vi "ADIS16448 Loop.vi"(8 "error in":errorcluster) -> ()   [LabVIEW 2019]
uses:
  Typedef/ADIS16448 Device Reference.ctl
  Typedef/ADIS16448 Hardware Configuration.ctl
  <vilib>/Rock Robotics/WPI/SPI/WPI_SPIMode.ctl
  <vilib>/Rock Robotics/SystemInterfaces/DIO/FPGA_DIOChannel.ctl
  <vilib>/Rock Robotics/SystemInterfaces/spilib/spi_bus.ctl
  Typedef/ADIS16448 Status.ctl
  Typedef/ADIS16448 Data.ctl
  Typedef/ADIS16448 Process.ctl
  Typedef/ADIS16448 Command Type.ctl
  <vilib>/Rock Robotics/SystemInterfaces/CounterEncoderSourceConvertion/FPGA_CounterEncoderSourceConvertionLVSourceType.ctl
  <vilib>/Rock Robotics/SystemInterfaces/DIO/FPGA_DIODigitalSourceChannel.ctl
  <vilib>/Rock Robotics/SystemInterfaces/AnalogTrigger/FPGA_AnalogTriggerIndex.ctl
  <vilib>/Rock Robotics/SystemInterfaces/AnalogTrigger/FPGA_AnalogTriggerOutType.ctl
  Typedef/ADIS16448 Loop State.ctl
  Typedef/ADIS16448 Loop Data.ctl
  <vilib>/Rock Robotics/WPI/SPI/WPI_SPIDevRef.ctl
  Typedef/ADIS16448 Register.ctl
  Typedef/ADIS16448 Call Buffer Cmd.ctl
  ADIS16448 Loop Update Globals.vi
  ADIS16448 Globals.vi
  <vilib>/Rock Robotics/WPI/Counter/WPI_CounterDigitalInputToDigitalSource.vi
  <vilib>/Rock Robotics/WPI/SPI/WPI_SPIWrite.vi
  <vilib>/Rock Robotics/WPI/SPI/WPI_SPIRead.vi
  <vilib>/Rock Robotics/WPI/ThirdParty/JAS_Junk/TrajLib/Trajectory_Library.lvlib
panel:
  in  "Use Register Read Mode":bool=TRUE
  in  "Calibration Time":i32
  in  "element":T1
  in  "ADIS16448DevRef":T2={"DevStatus"={"status"=FALSE, "code"=0, "source"=""}, "Hardware Config"={"SPI Clock Rate (Hz)"=1000000.0, "IMU SPI Mode (3)"=enum."Mode 3 (Clk Idle High,Sample on Trailing)", "IMU Reset Pin"=enum."SPI Port CS2", "IMU SPI Bus"=enum."SPI On-Board, CS0", "IMU Data Ready Pin"=enum."SPI Port CS1", "Stall Config"={"Pow2BytesPerRead"=255, "StallTicks"=640, "CsToSclkTicks"=5}, "IMU Status LED Pin"=enum."DIO MXP 9"}, "Calibration Complete"=refnum, "Status FIFO"=refnum, "Last Value Reference"=refnum, "Sychronous Process VI"=refnum, "Cmd FIFO"=refnum, "Source"={"DevStatus"={"status"=FALSE, "code"=0, "source"=""}, "AnalogTriggerMode?"=FALSE, "DigitalMode"={"DIO Channel"=enum."Disabled"}, "AnalogTriggerMode"={"AnalogTriggerIndex"=enum."Trig 0", "OutputType"=enum."InWindow"}}, "Data FIFO"=refnum, "IMU Status LED Pin"=enum."DIO MXP 9", "Calibration Time"=5}
  in  "Main Name":string
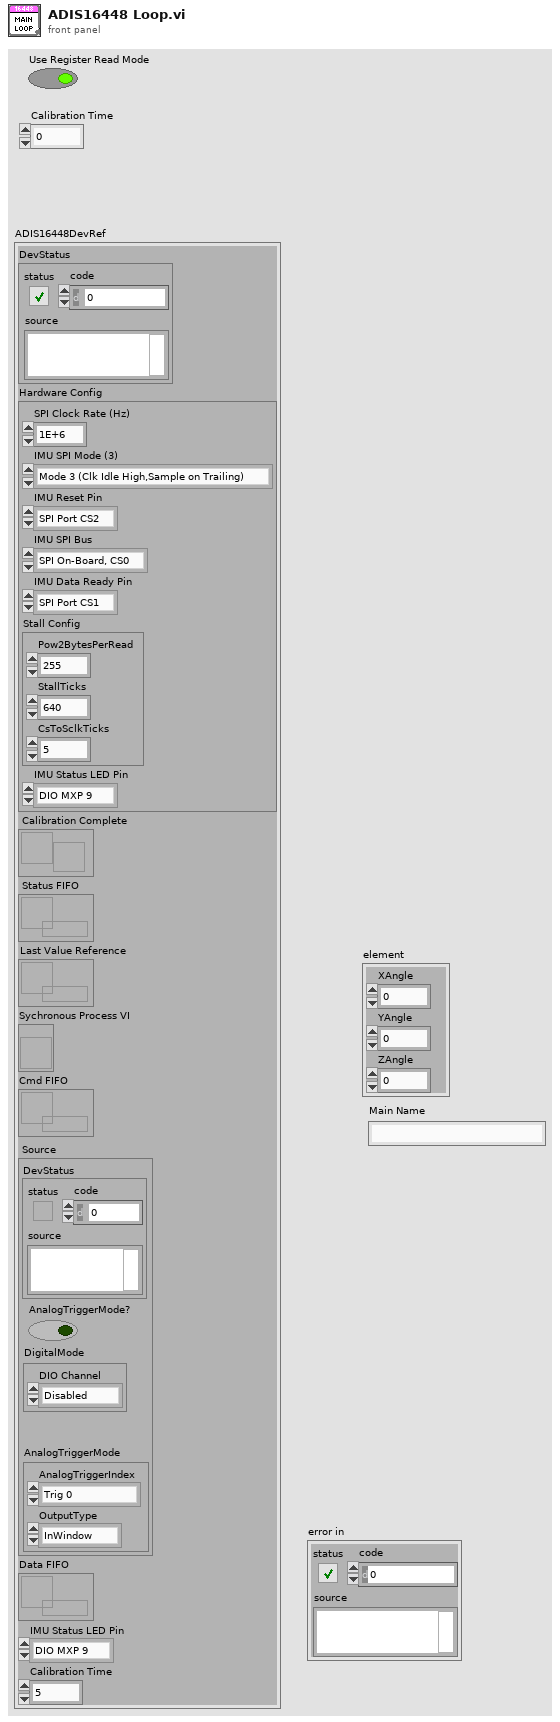
[diagram p1: front panel]
types:
  T1 = typedef "ADIS16448 Data.ctl" = cluster{"XAngle":dbl, "YAngle":dbl, "ZAngle":dbl}
  T2 = typedef "ADIS16448 Device Reference.ctl" = cluster{"DevStatus":errorcluster, "Hardware Config":T3, "Calibration Complete":refnum<notifier>, "Status FIFO":refnum<k33>, "Last Value Reference":refnum<data-value>, "Sychronous Process VI":T7, "Cmd FIFO":refnum<k33>, "Source":T8, "Data FIFO":refnum<k33>, "IMU Status LED Pin":T5, "Calibration Time":u32}
  T3 = typedef "ADIS16448 Hardware Configuration.ctl" = cluster{"SPI Clock Rate (Hz)":dbl, "IMU SPI Mode (3)":T4, "IMU Reset Pin":T5, "IMU SPI Bus":T6, "IMU Data Ready Pin":T5, "Stall Config":cluster{"Pow2BytesPerRead":u8, "StallTicks":u16, "CsToSclkTicks":u8}, "IMU Status LED Pin":T5}
  T4 = typedef "WPI_SPIMode.ctl" = enum16{"Mode 0 (Clk Idle Low,Sample on Leading)", "Mode 1 (Clk Idle Low,Sample on Trailing)", "Mode 2 (Clk Idle High,Sample on Leading)", "Mode 3 (Clk Idle High,Sample on Trailing)"}
  T5 = typedef "FPGA_DIOChannel.ctl" = enum8{"DIO 0", "DIO 1", "DIO 2", "DIO 3", "DIO 4", "DIO 5", "DIO 6", "DIO 7", "DIO 8", "DIO 9", "DIO MXP 0", "DIO MXP 1", "DIO MXP 2", "DIO MXP 3", "DIO MXP 4", "DIO MXP 5", "DIO MXP 6", "DIO MXP 7", "DIO MXP 8", "DIO MXP 9", "DIO MXP 10", "DIO MXP 11", "DIO MXP 12", "DIO MXP 13", "DIO MXP 14", "DIO MXP 15", "SPI Port CS1", "SPI Port CS2", "SPI Port CS3", "SPI Port MISO", "SPI Port MOSI", "Invalid"}
  T6 = typedef "spi_bus.ctl" = enum16{"SPI On-Board, CS0", "SPI On-Board, CS1", "SPI On-Board, CS2", "SPI On-Board, CS3", "SPI MXP", "Invalid"}
  T7 = typedef "ADIS16448 Process.ctl" = refnum<vi>
  T8 = typedef "FPGA_CounterEncoderSourceConvertionLVSourceType.ctl" = cluster{"DevStatus":errorcluster, "AnalogTriggerMode?":bool, "DigitalMode":cluster{"DIO Channel":T9}, "AnalogTriggerMode":cluster{"AnalogTriggerIndex":T10, "OutputType":T11}}
  T9 = typedef "FPGA_DIODigitalSourceChannel.ctl" = enum8{"DIO 0", "DIO 1", "DIO 2", "DIO 3", "DIO 4", "DIO 5", "DIO 6", "DIO 7", "DIO 8", "DIO 9", "DIO MXP 0", "DIO MXP 1", "DIO MXP 2", "DIO MXP 3", "DIO MXP 4", "DIO MXP 5", "DIO MXP 6", "DIO MXP 7", "DIO MXP 8", "DIO MXP 9", "DIO MXP 10", "DIO MXP 11", "DIO MXP 12", "DIO MXP 13", "DIO MXP 14", "DIO MXP 15", "SPI Port CS1", "SPI Port CS2", "SPI Port CS3", "SPI Port MISO", "SPI Port MOSI", "Disabled"}
  T10 = typedef "FPGA_AnalogTriggerIndex.ctl" = enum8{"Trig 0", "Trig 1", "Trig 2", "Trig 3", "Trig 4", "Trig 5", "Trig 6", "Trig 7", "Invalid"}
  T11 = typedef "FPGA_AnalogTriggerOutType.ctl" = enum16{"InWindow", "TriggerState", "Rising", "Falling"}
  T12 = typedef "ADIS16448 Register.ctl" = u8
  T13 = typedef "ADIS16448 Loop State.ctl" = enum16{"Default", "Error", "***Initialization***", "Reset", "Register DR Source", "Start SPI", "Write Config", "Init Auto SPI", "***Calibration***", "Calibrate", "Finish Cal", "***Operation***", "Run", "Process", "Run Cmds", "Run_Alt", "Run_Cmds_Alt", "Cal_Init_Alt", "Cal_Alt"}
  T14 = typedef "ADIS16448 Loop Data.ctl" = cluster{"SPIDevRef":T15, "Data Counter":u16, "Reset":bool, "Digital Source":T8, "Bytes Per Sample":u32, "Data":dbl[], "ADIS16448DevRef":T2, "TimeStampPrev":u32, "Sensor to Robot Rotation":dbl[][], "AutoSPI Active?":bool, "Offsets":dbl[], "Offset Counter":i32, "Data Header":u8[], "Zero Byte Count":u8, "Running Offset":dbl[], "CalSamplesAlt":i32, "CalCountAlt":i32}
  T15 = typedef "WPI_SPIDevRef.ctl" = cluster{"DevStatus":errorcluster, "Handle":i32, "SPI Bus":T6}
  T16 = typedef "ADIS16448 Status.ctl" = cluster{"Calibrated?":bool, "IMU Detected?":bool}
  T17 = typedef "ADIS16448 Call Buffer Cmd.ctl" = enum16{"Add Item ", "Calculate"}
  T18 = typedef "ADIS16448 Command Type.ctl" = cluster{"Command":enum16{"None", "Reset", "Rewrite Config", "Start Recal", "Recalibrate", "Recal Complete", "Exit Auto SPI", "Start Auto SPI", "Configure Cal"}, "Data":u32}
  T19 = typedef "WPI_DigitalOutputDevRef.ctl" = cluster{"DIO Channel":T5, "DevStatus":errorcluster}
  T20 = typedef "WPI_DigitalInputDevRef.ctl" = cluster{"DevStatus":errorcluster, "DIO Channel":T5}
  T21 = cluster{"Pow2BytesPerRead":u8, "StallTicks":u16, "CsToSclkTicks":u8}
  T22 = enum16{"None", "Reset", "Rewrite Config", "Start Recal", "Recalibrate", "Recal Complete", "Exit Auto SPI", "Start Auto SPI", "Configure Cal"}
  T23 = enum32{"Bad", "Idle", "Run top level", "Running"}
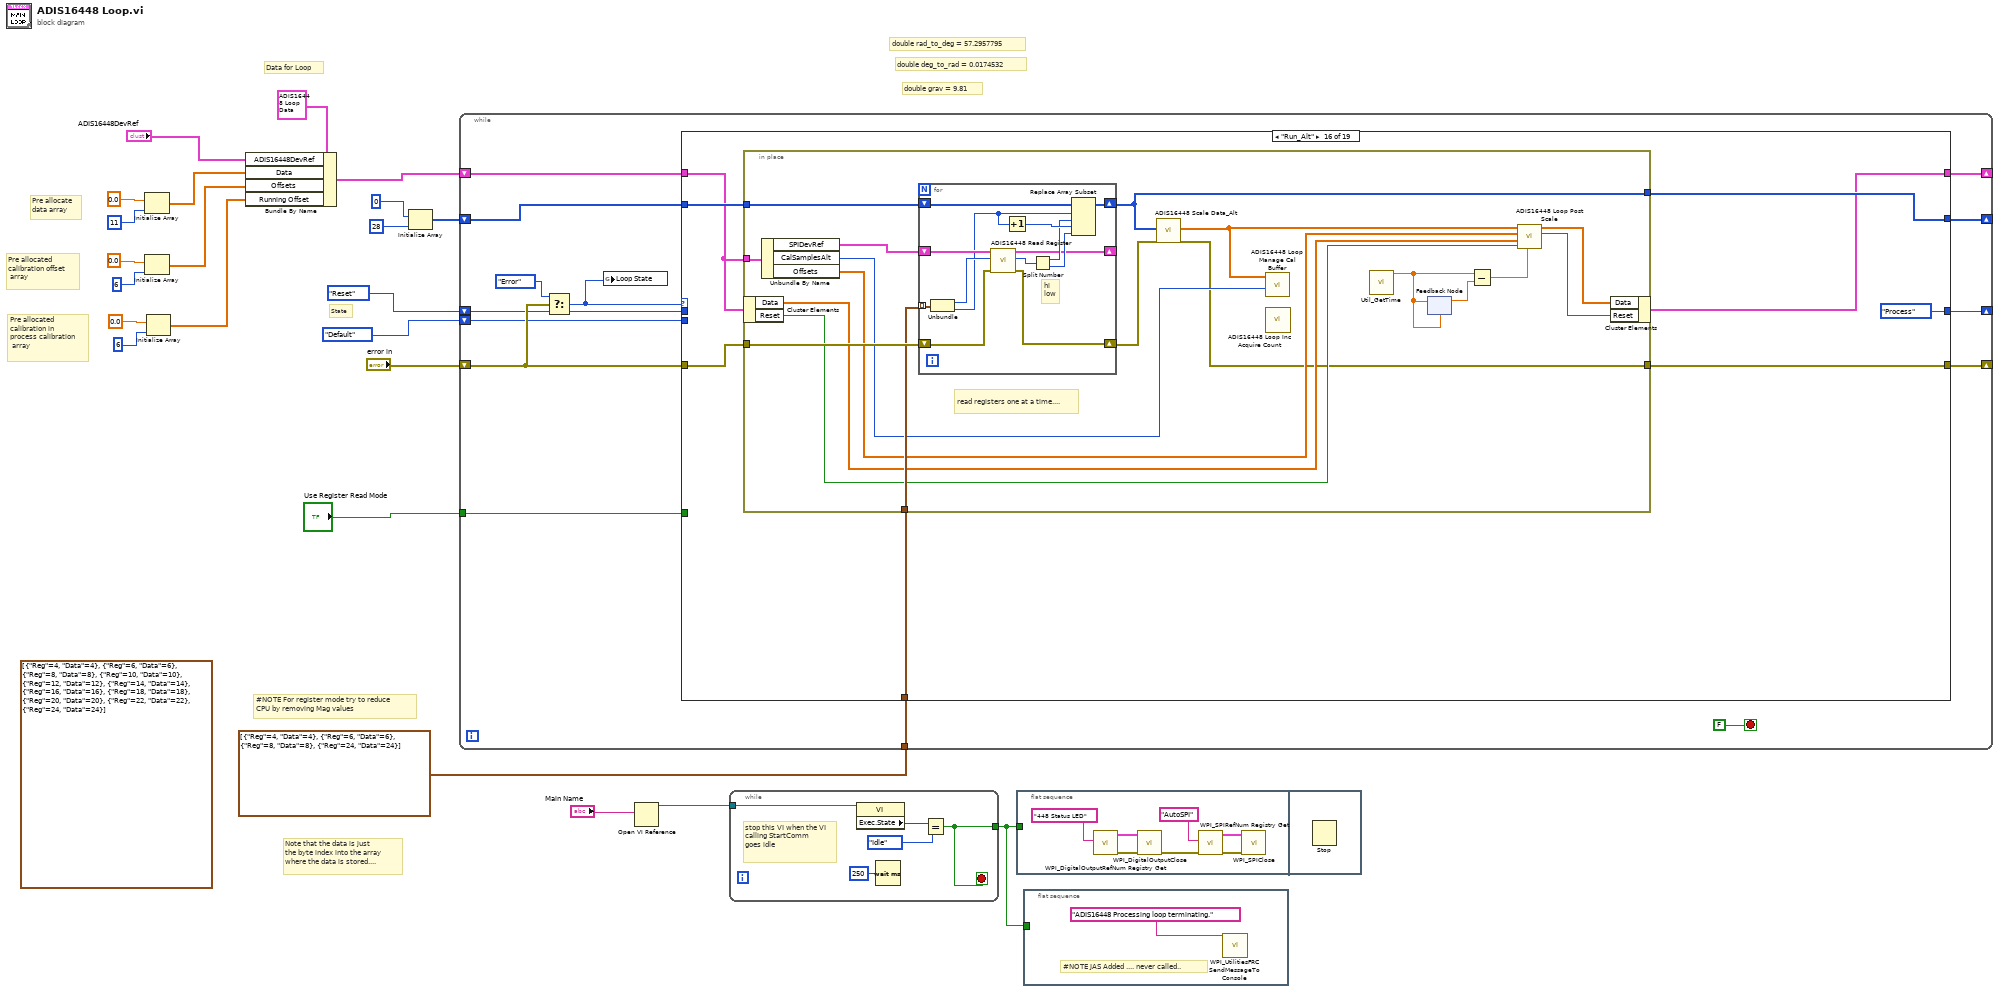
[diagram p0: block diagram]
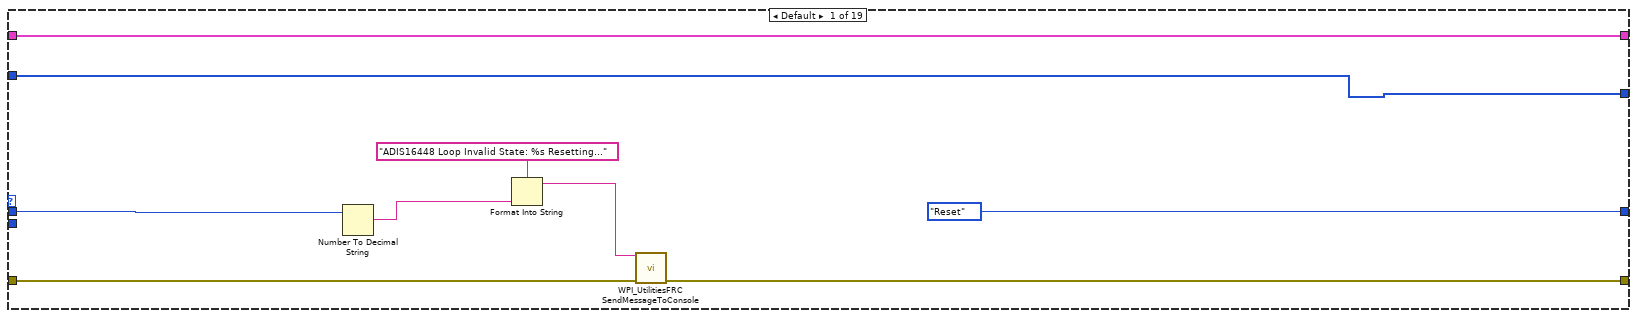
[diagram p2: hidden frame]
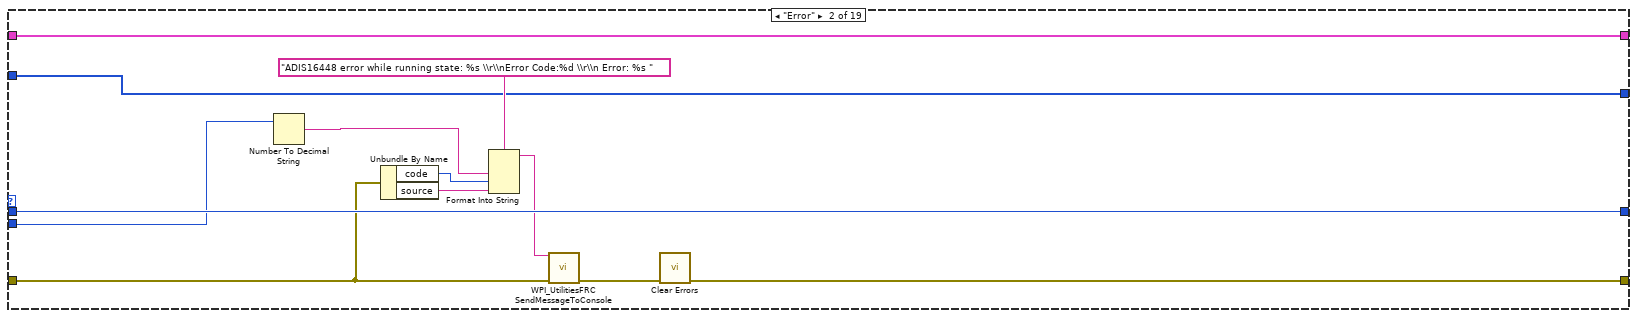
[diagram p3: hidden frame]
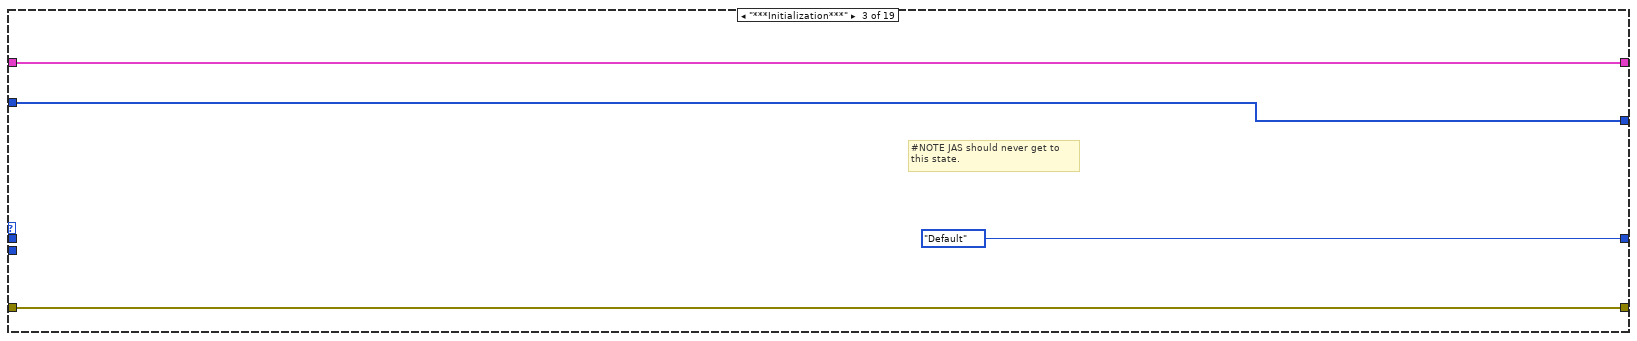
[diagram p4: hidden frame]
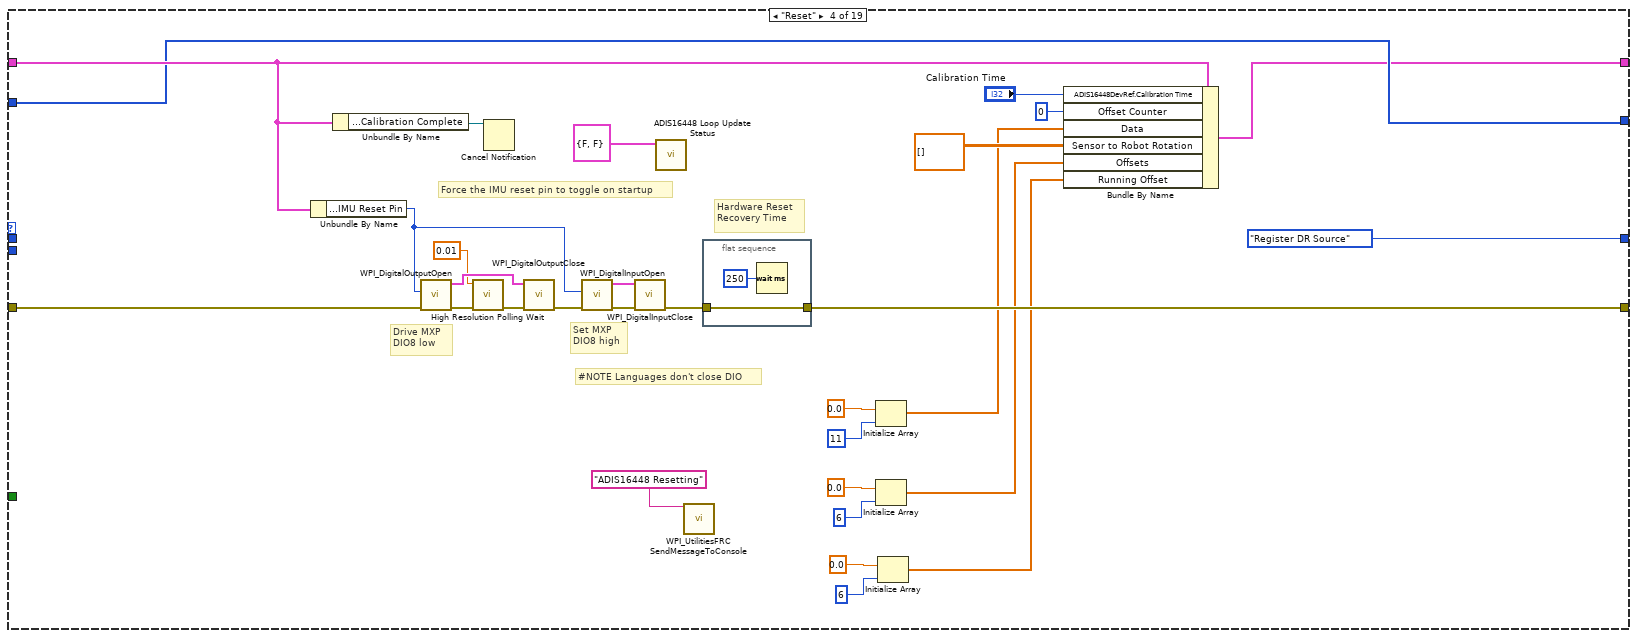
[diagram p5: hidden frame]
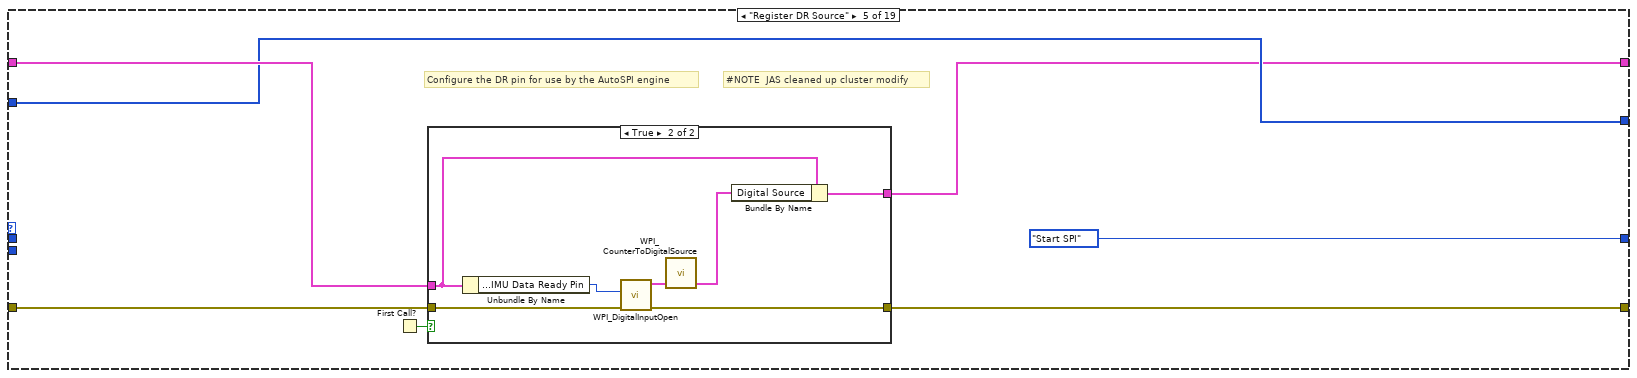
[diagram p6: hidden frame]
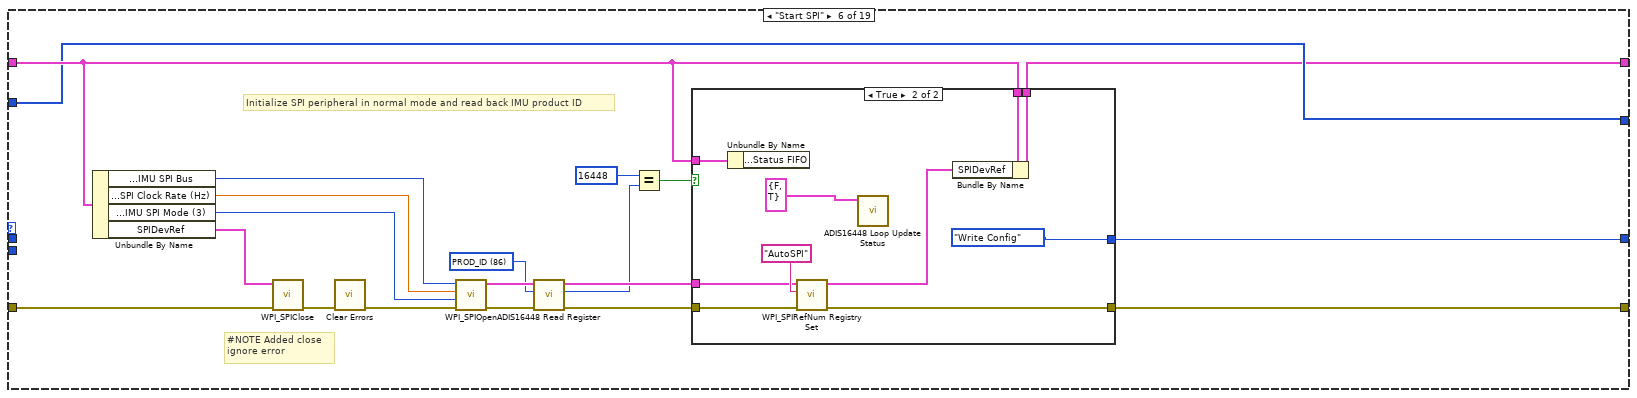
[diagram p8: hidden frame]
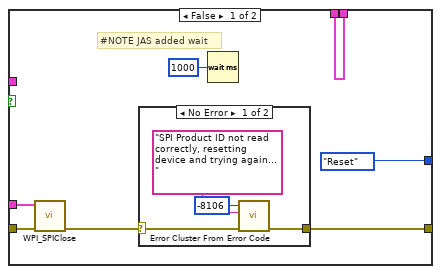
[diagram p9: hidden frame]
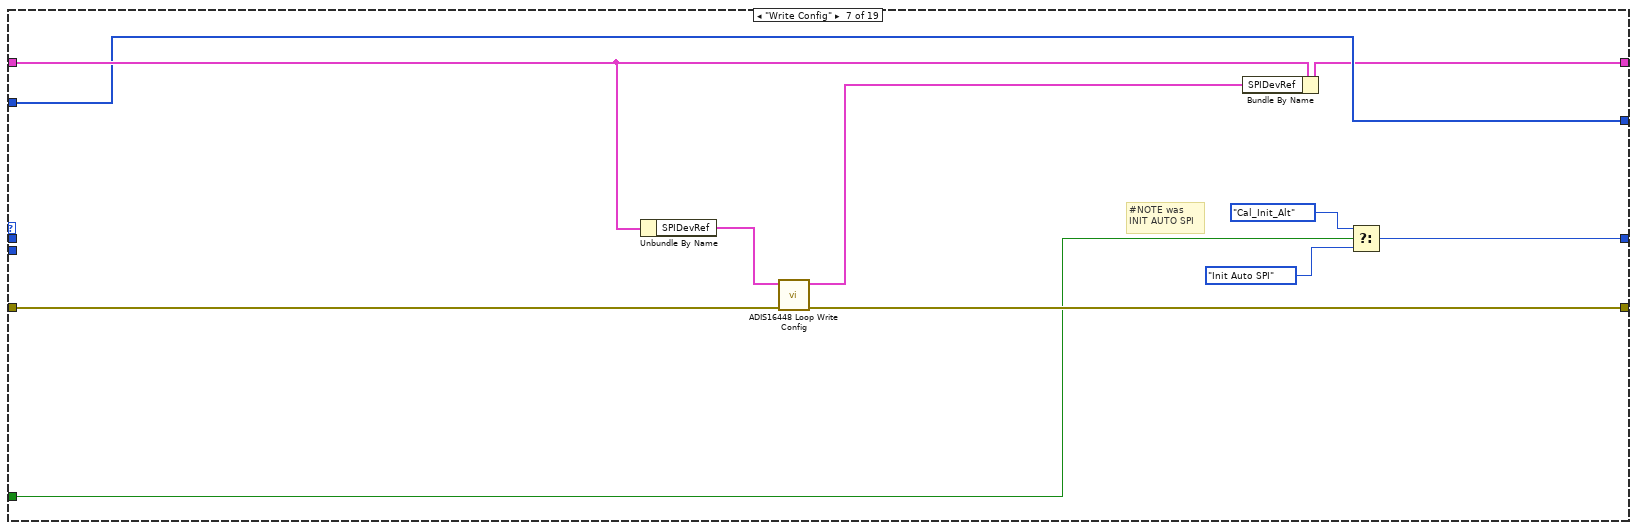
[diagram p11: hidden frame]
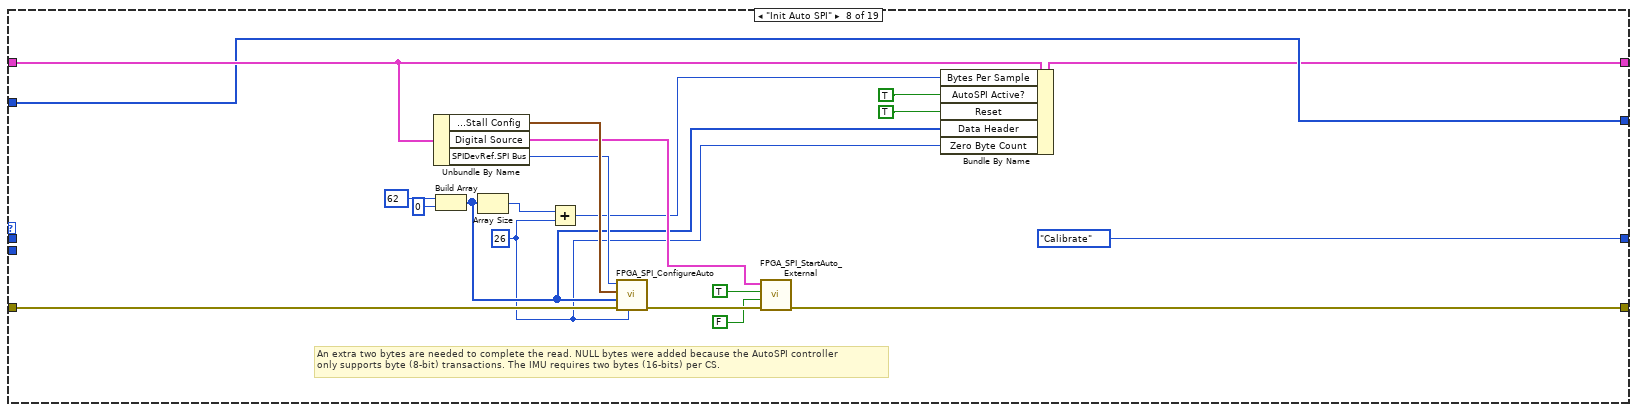
[diagram p12: hidden frame]
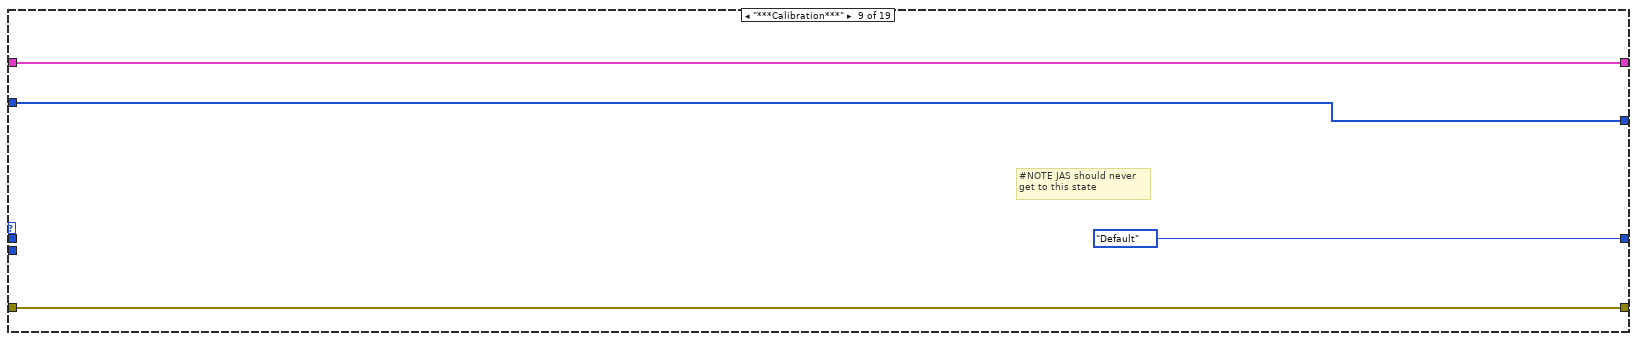
[diagram p13: hidden frame]
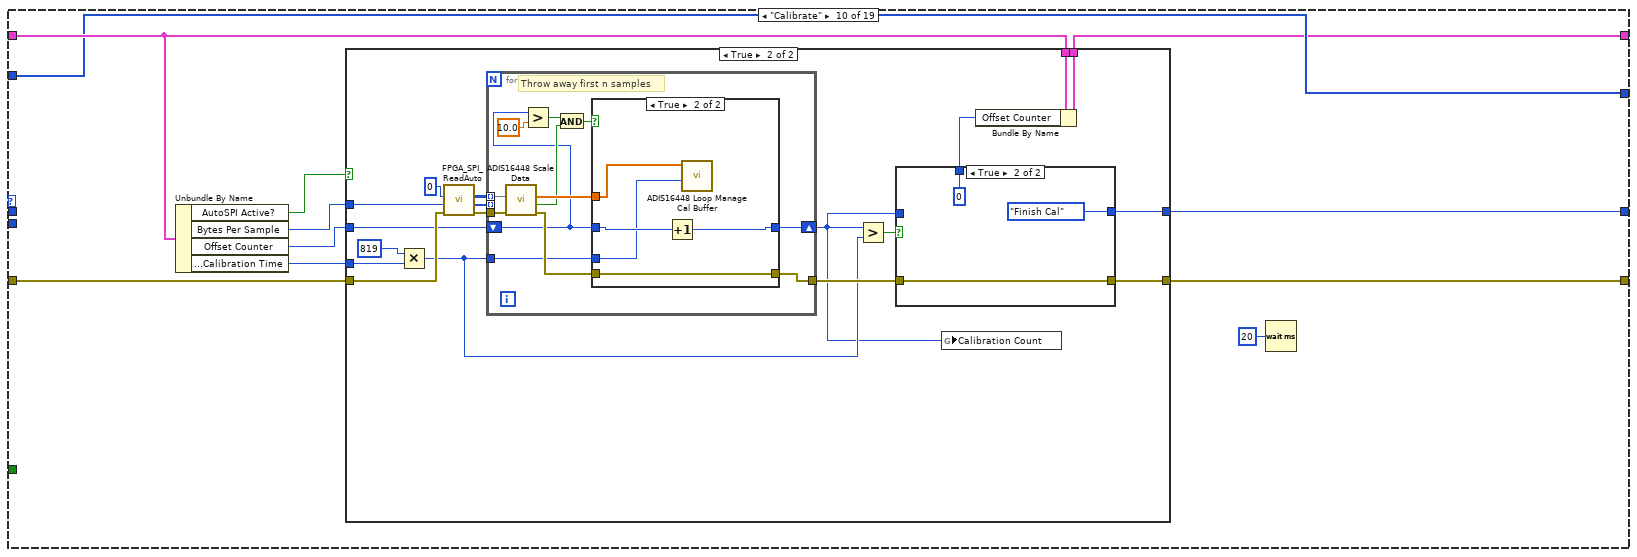
[diagram p14: hidden frame]
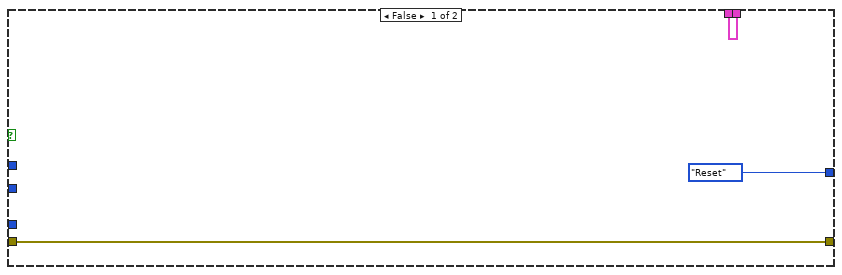
[diagram p15: hidden frame]
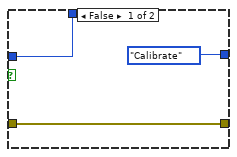
[diagram p16: hidden frame]
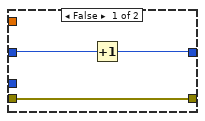
[diagram p17: hidden frame]
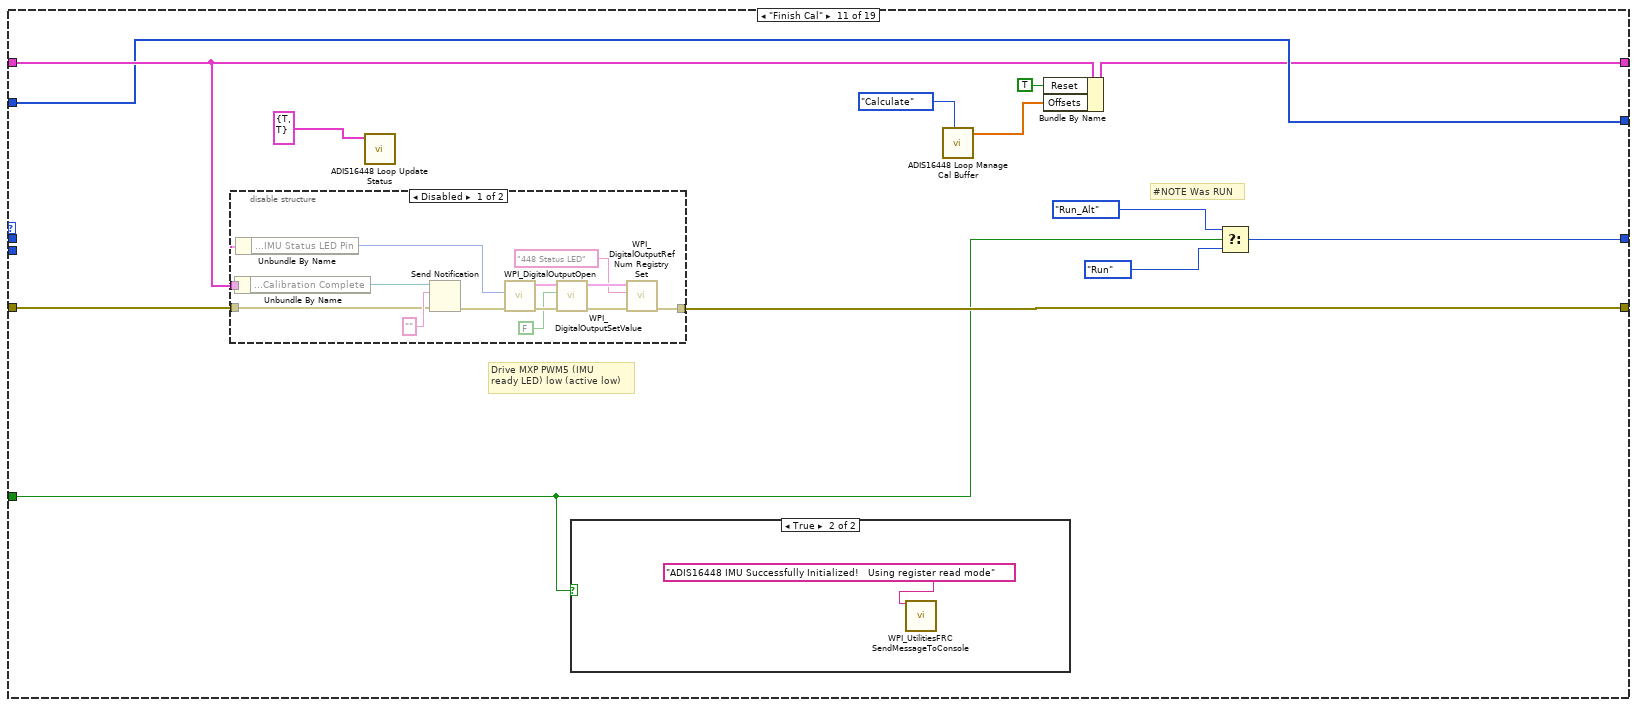
[diagram p18: hidden frame]
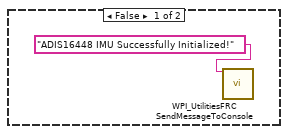
[diagram p19: hidden frame]
diagram:
  (unwired) cluster{"Reg":T12, "Data":u16}[] [{"Reg"=4, "Data"=4}, {"Reg"=6, "Data"=6}, {"Reg"=8, "Data"=8}, {"Reg"=10, "Data"=10}, {"Reg"=12, "Data"=12}, {"Reg"=14, "Data"=14}, {"Reg"=16, "Data"=16}, {"Reg"=18, "Data"=18}, {"Reg"=20, "Data"=20}, {"Reg"=22, "Data"=22}, {"Reg"=24, "Data"=24}]
  # "Note that the data is just\nthe byte index into the array\nwhere the data is stored...."
  # "#NOTE For register mode try to reduce\nCPU by removing Mag values"
  # "Pre allocated\ncalibration in\nprocess calibration\n array"
  # "Pre allocated\ncalibration offset\n array"
  # "Pre allocate\ndata array"
  # "Data for Loop"
  # "State"
  # "double grav = 9.81"
  # "double deg_to_rad = 0.0174532"
  # "double rad_to_deg = 57.2957795"
  n1 = Initialize Array(0.0, 11 ("dimension size")) -> (w9:dbl[])
  n2 = Initialize Array(0.0, 6 ("dimension size")) -> (w6:dbl[])
  n3 = Initialize Array(0.0, 6 ("dimension size")) -> (w2:dbl[])
  n4 = Bundle By Name(cluster=T14 {"SPIDevRef"={"DevStatus"={"status"=FALSE, "code"=0, "source"=""}, "Handle"=0, "SPI Bus"=enum."SPI On-Board, CS0"}, "Data Counter"=0, "Reset"=FALSE, "Digital Source"={"DevStatus"={"status"=FALSE, "code"=0, "source"=""}, "AnalogTriggerMode?"=FALSE, "DigitalMode"={"DIO Channel"=enum."DIO 1"}, "AnalogTriggerMode"={"AnalogTriggerIndex"=enum."Trig 0", "OutputType"=enum."InWindow"}}, "Bytes Per Sample"=0, "Data"=[0.0, 0.0, 0.0, 0.0, 0.0, 0.0, 0.0, 0.0], "ADIS16448DevRef"={"DevStatus"={"status"=FALSE, "code"=0, "source"=""}, "Hardware Config"={"SPI Clock Rate (Hz)"=1000000.0, "IMU SPI Mode (3)"=enum."Mode 3 (Clk Idle High,Sample on Trailing)", "IMU Reset Pin"=enum."SPI Port CS2", "IMU SPI Bus"=enum."SPI On-Board, CS0", "IMU Data Ready Pin"=enum."SPI Port CS1", "Stall Config"={"Pow2BytesPerRead"=255, "StallTicks"=640, "CsToSclkTicks"=5}, "IMU Status LED Pin"=enum."DIO MXP 9"}, "Calibration Complete"=refnum, "Status FIFO"=refnum, "Last Value Reference"=refnum, "Sychronous Process VI"=refnum, "Cmd FIFO"=refnum, "Source"={"DevStatus"={"status"=FALSE, "code"=0, "source"=""}, "AnalogTriggerMode?"=FALSE, "DigitalMode"={"DIO Channel"=enum."Disabled"}, "AnalogTriggerMode"={"AnalogTriggerIndex"=enum."Trig 0", "OutputType"=enum."InWindow"}}, "Data FIFO"=refnum, "IMU Status LED Pin"=enum."DIO MXP 9", "Calibration Time"=5}, "TimeStampPrev"=0, "Sensor to Robot Rotation"=[], "AutoSPI Active?"=TRUE, "Offsets"=[0.0, 0.0, 0.0, 0.0, 0.0, 0.0, 0.0, 0.0], "Offset Counter"=0, "Data Header"=[], "Zero Byte Count"=0, "Running Offset"=[0.0, 0.0, 0.0, 0.0, 0.0, 0.0, 0.0, 0.0], "CalSamplesAlt"=0, "CalCountAlt"=0}, "ADIS16448DevRef"="ADIS16448DevRef", "Data"=w9, "Offsets"=w6, "Running Offset"=w2) -> (w19:T14)
  n5 = Initialize Array(u8 0, 28 ("dimension size")) -> (w12:u8[])
  n6 = while {
    shift-right: [w34] -> _
    shift-left: ADIS16448_Loop_State."Reset" -> [w32]
    shift-right: [w24] -> _
    shift-left: w19 -> [w36]
    shift-right: [w35] -> _
    shift-left: "error in" -> [w33]
    shift-left: ADIS16448_Loop_State."Default" -> [w30]
    shift-right: [w27] -> _
    shift-left: w12 -> [w28]
    tunnel: cluster{"Reg":T12, "Data":u16}[] [{"Reg"=4, "Data"=4}, {"Reg"=6, "Data"=6}, {"Reg"=8, "Data"=8}, {"Reg"=24, "Data"=24}] -> [w26]
    tunnel: "Use Register Read Mode" -> [w25]
    stop <- FALSE stop-if-true
    n7 = Select(t=ADIS16448_Loop_State."Error", s=w33, f=w32) -> (s? t:f=w29:T13)
    n8 = global write "ADIS16448 Globals.vi" "Loop State"(w29) -> ()
    n9 = case shown="\"Run_Alt\"" w29 {
      tunnel: w36 -> [w38 w47 w59 w89 w98 w122 w161 w178 w184 w191 w256 w274 w281 w335 w364 w489 w530 w676 w687]
      tunnel: w33 -> [w46 w55 w62 w83 w100 w117 w162 w182 w187 w197 w257 w277 w283 w346 w370 w495 w531 w677 w702]
      tunnel: [w45 w56 w62 w91 w99 w126 w159 w166 w187 w196 w255 w277 w282 w345 w369 w493 w529 w677 w683] -> w35
      tunnel: [ADIS16448_Loop_State."Reset" w58 ADIS16448_Loop_State."Default" ADIS16448_Loop_State."Register DR Source" ADIS16448_Loop_State."Start SPI" w127 w156 ADIS16448_Loop_State."Calibrate" ADIS16448_Loop_State."Default" w192 w252 ADIS16448_Loop_State."Default" ADIS16448_Loop_State."Process" w340 w362 ADIS16448_Loop_State."Process" w528 ADIS16448_Loop_State."Cal_Alt" w698] -> w34
      tunnel: w32 -> [w41 w58 _ _ _ _ _ _ _ _ _ _ _ _ _ _ _ _ _]
      tunnel: w30 -> [_ w49 _ _ _ _ _ _ _ _ _ _ _ _ _ _ _ _ _]
      tunnel: w28 -> [w39 w48 w60 w74 w96 w112 w158 w165 w185 w189 w254 w275 w279 w342 w361 w492 w539 w670 w695]
      tunnel: [w39 w48 w60 w74 w96 w112 w158 w165 w185 w189 w254 w275 w279 w342 w361 w491 w539 w670 w693] -> w27
      tunnel: w26 -> [_ _ _ _ _ _ _ _ _ _ _ _ _ _ _ w490 _ _ w689]
      tunnel: w25 -> [_ _ _ _ _ _ w154 _ _ _ w250 _ _ w338 _ _ _ _ _]
      tunnel: [w38 w47 w59 w63 w95 w111 w153 w164 w184 w188 w246 w274 w278 w335 w360 w488 w527 w669 w686] -> w24
      frame Default {
        n10 = Number To Decimal String(number=w41) -> (decimal integer string=w40:string)  [unwired: 1 in]
        n11 = Format Into String(format string="ADIS16448 Loop Invalid State: %s Resetting...", w40) -> (resulting string=w44:string)  [unwired: 2 in, 1 out]
        n12 = call <vilib>:"WPI_UtilitiesFRC SendMessageToConsole.vi"("Message"=w44, "error in (no error)"=w46) -> ("error out"=w45:errorcluster)  [unwired: 13 in]
      }
      frame "Error" {
        n13 = Number To Decimal String(number=w49) -> (decimal integer string=w50:string)  [unwired: 1 in]
        n14 = Unbundle By Name(w55) -> ("code"=w52:i32, "source"=w51:string)
        n15 = Format Into String(format string="ADIS16448 error while running state: %s \\r\\nError Code:%d \\r\\n Error: %s ", w50, w52, w51) -> (resulting string=w54:string)  [unwired: 2 in, 1 out]
        n16 = call <vilib>:"WPI_UtilitiesFRC SendMessageToConsole.vi"("Message"=w54, "error in (no error)"=w55) -> ("error out"=w57:errorcluster)  [unwired: 13 in]
        n17 = call <vilib>:"Clear Errors.vi"("error in (no error)"=w57) -> ("error out"=w56:errorcluster)  [unwired: 5 in, 1 out]
      }
      frame "***Initialization***" {
        # "#NOTE JAS should never get to \nthis state."
      }
      frame "Reset" {
        # "Set MXP \nDIO8 high"
        # "Drive MXP \nDIO8 low"
        # "#NOTE Languages don't close DIO"
        # "Hardware Reset Recovery Time"
        # "Force the IMU reset pin to toggle on startup"
        n18 = Unbundle By Name(w89) -> ("ADIS16448DevRef.Hardware Config.IMU Reset Pin"=w79:T5)
        n19 = Unbundle By Name(w89) -> ("ADIS16448DevRef.Calibration Complete"=w90:refnum<notifier>)
        n20 = call <vilib>:"WPI_DigitalOutputOpen.vi"("error in (no error)"=w83, "DIO Channel"=w79) -> ("error out"=w81:errorcluster, "DigitalOutputDevRef"=w88:T19)  [unwired: 8 in]
        n21 = call <vilib>:"High Resolution Polling Wait.vi"("error in (no error)"=w81, "seconds to wait"=0.01) -> ("error out"=w82:errorcluster)  [unwired: 9 in]
        n22 = Cancel Notification(0:w90) -> ()  [unwired: 1 in, 3 out]
        n23 = call <vilib>:"WPI_DigitalOutputClose.vi"("error in (no error)"=w82, "DigitalOutputDevRef"=w88) -> ("error out"=w85:errorcluster)  [unwired: 9 in]
        n24 = call <vilib>:"WPI_DigitalInputOpen.vi"("error in (no error)"=w85, "DIO Channel"=w79) -> ("error out"=w86:errorcluster, "DigitalInputDevRef"=w87:T20)  [unwired: 8 in]
        n25 = call <vilib>:"WPI_DigitalInputClose.vi"("error in (no error)"=w86, "DigitalInputDevRef"=w87) -> ("error out"=w84:errorcluster)  [unwired: 9 in]
        n26 = call "ADIS16448 Loop Update Status.vi"("ADIS16448 Status"=T16 {"Calibrated?"=FALSE, "IMU Detected?"=FALSE} ("element")) -> ()  [unwired: 10 in, 1 out]
        n27 = call <vilib>:"WPI_UtilitiesFRC SendMessageToConsole.vi"("Message"="ADIS16448 Resetting" ("format string")) -> ()  [unwired: 14 in, 1 out]
        n28 = flat-sequence {
          tunnel: [w94] -> w91
          tunnel: w84 -> [w94]
          frame #0 {
            n29 = Wait (ms)(milliseconds to wait=u32 250) -> ()  [unwired: 1 out]
          }
        }
        n30 = Initialize Array(0.0, 11 ("dimension size")) -> (w67:dbl[])
        n31 = Initialize Array(0.0, 6 ("dimension size")) -> (w66:dbl[])
        n32 = Initialize Array(0.0, 6 ("dimension size")) -> (w65:dbl[])
        n33 = Bundle By Name(cluster=w89, "ADIS16448DevRef.Calibration Time"="Calibration Time", "Offset Counter"=0, "Data"=w67, "Sensor to Robot Rotation"=dbl[][] [], "Offsets"=w66, "Running Offset"=w65) -> (w63:T14)
      }
      frame "Register DR Source" {
        # "#NOTE  JAS cleaned up cluster modify"
        # "Configure the DR pin for use by the AutoSPI engine"
        n34 = First Call?() -> (First Call?: T/F=w97:bool)
        n35 = case shown="True" w97 {
          tunnel: w100 -> [w103 w110]
          tunnel: w98 -> [w102 w106]
          tunnel: [w103 w107] -> w99
          tunnel: [w102 w104] -> w95
          frame False {
          }
          frame True {
            n36 = Unbundle By Name(w106) -> ("ADIS16448DevRef.Hardware Config.IMU Data Ready Pin"=w108:T5)
            n37 = call <vilib>:"WPI_DigitalInputOpen.vi"("error in (no error)"=w110, "DIO Channel"=w108) -> ("error out"=w107:errorcluster, "DigitalInputDevRef"=w109:T20)  [unwired: 8 in]
            n38 = call-poly <vilib>:"WPI_CounterToDigitalSource.vi"("DigitalInputDevRef"=w109) -> ("Digital Source"=w105:T8)  [unwired: 6 in]
            n39 = Bundle By Name(cluster=w106, "Digital Source"=w105) -> (w104:T14)
          }
        }
      }
      frame "Start SPI" {
        w121 = T12 86 items=["FLASH_CNT"=0, "Reserved 1"=2, "XGYRO_OUT"=4, "YGYRO_OUT"=6, "ZGYRO_OUT"=8, "XACCL_OUT"=10, "YACCL_OUT"=12, "ZACCL_OUT"=14, "XMAGN_OUT"=16, "YMAGN_OUT"=18, "ZMAGN_OUT"=20, "BARO_OUT"=22, "TEMP_OUT"=24, "XGYRO_OFF"=26, "YGYRO_OFF"=28, "ZGYRO_OFF"=30, "XACCL_OFF"=32, "YACCL_OFF"=34, "ZACCL_OFF"=36, "XMAGN_HIC"=38, "YMAGN_HIC"=40, "ZMAGN_HIC"=42, "XMAGN_SIC"=44, "YMAGN_SIC"=46, "ZMAGN_SIC"=48, "GPIO_CTRL"=50, "MSC_CTRL"=52, "SMPL_PRD"=54, "SENS_AVG"=56, "SEQ_CNT"=58, "DIAG_STAT"=60, "GLOB_CMD"=62, "ALM_MAG1"=64, "ALM_MAG2"=66, "ALM_SMPL1"=68, "ALM_SMPL2"=70, "ALM_CTRL"=72, "Reserved 2"=74, "Reserved 3"=76, "Reserved 4"=78, "Reserved 5"=80, "LOT_ID1"=82, "LOT_ID2"=84, "PROD_ID"=86, "SERIAL_NUM"=88] ("ADIS16448 Register")
        # "#NOTE Added close\nignore error"
        # "Initialize SPI peripheral in normal mode and read back IMU product ID"
        n40 = Unbundle By Name(w122) -> ("ADIS16448DevRef.Hardware Config.IMU SPI Bus"=w114:T6, "ADIS16448DevRef.Hardware Config.SPI Clock Rate (Hz)"=w128:dbl, "ADIS16448DevRef.Hardware Config.IMU SPI Mode (3)"=w129:T4, "SPIDevRef"=w113:T15)
        n41 = call <vilib>:"WPI_SPIClose.vi"("error in (no error)"=w117, "SPIDevRef"=w113) -> ("error out"=w116:errorcluster)  [unwired: 9 in]
        n42 = call <vilib>:"Clear Errors.vi"("error in (no error)"=w116) -> ("error out"=w115:errorcluster)  [unwired: 5 in, 1 out]
        n43 = call <vilib>:"WPI_SPIOpen.vi"("error in"=w115, "Mode (3)"=w129, "Clock Rate (Hz)"=w128, "SPI Bus"=w114) -> ("error out"=w125:errorcluster, "SPIDevRef"=w124:T15)  [unwired: 6 in]
        n44 = call "ADIS16448 Read Register.vi"("error in (no error)"=w125, "ADIS16448 Register"=w121, "SPIDevRef in"=w124) -> ("error out"=w119:errorcluster, "Register Value"=w118:u16, "SPIDevRef out"=w120:T15)  [unwired: 6 in]
        n45 = Equal?(x=u16 16448 ("y"), y=w118) -> (x = y?=w130:bool)
        n46 = case shown="True" w130 {
          tunnel: [ADIS16448_Loop_State."Reset" ADIS16448_Loop_State."Write Config"] -> w127
          tunnel: w122 -> [w136 w151]
          tunnel: [w136 w150] -> w111
          tunnel: [w135 w145] -> w126
          tunnel: w119 -> [w134 w146]
          tunnel: w120 -> [w133 w147]
          tunnel: w122 -> [_ w144]
          frame False {
            # "#NOTE JAS added wait"
            n47 = call <vilib>:"WPI_SPIClose.vi"("error in (no error)"=w134, "SPIDevRef"=w133) -> ("error out"=w132:errorcluster)  [unwired: 9 in]
            n48 = case shown="No Error" w132 {
              selector: w132 -> [w140 w142]
              tunnel: [w141 w142] -> w135
              frame No Error {
                n49 = call <vilib>:"Error Cluster From Error Code.vi"("error in (no error)"=w140, "error message (\"\")"="SPI Product ID not read correctly, resetting device and trying again..." ("error message (\"\")"), "error code (0)"=-8106) -> ("error out"=w141:errorcluster)  [unwired: 6 in]
              }
              frame Error {
              }
            }
            n50 = Wait (ms)(milliseconds to wait=u32 1000) -> ()  [unwired: 1 out]
          }
          frame True {
            n51 = Unbundle By Name(w144) -> ()  [unwired: 1 out]
            n52 = call <vilib>:"WPI_SPIRefNum Registry Set.vi"("error in (no error)"=w146, "refnum name"="AutoSPI", "SPIDevRef"=w147) -> ("error out"=w145:errorcluster, "SPIDevRef"=w149:T15)  [unwired: 7 in]
            n53 = call "ADIS16448 Loop Update Status.vi"("ADIS16448 Status"=T16 {"Calibrated?"=FALSE, "IMU Detected?"=TRUE} ("element")) -> ()  [unwired: 10 in, 1 out]
            n54 = Bundle By Name(cluster=w151, "SPIDevRef"=w149) -> (w150:T14)
          }
        }
      }
      frame "Write Config" {
        # "#NOTE was\nINIT AUTO SPI"
        n55 = Unbundle By Name(w161) -> ("SPIDevRef"=w163:T15)
        n56 = call "ADIS16448 Loop Write Config.vi"("error in (no error)"=w162, "SPIDevRef"=w163) -> ("error out"=w159:errorcluster, "SPIDevRef out"=w160:T15)  [unwired: 8 in]
        n57 = Bundle By Name(cluster=w161, "SPIDevRef"=w160) -> (w153:T14)
        n58 = Select(t=ADIS16448_Loop_State."Cal_Init_Alt", s=w154, f=ADIS16448_Loop_State."Init Auto SPI") -> (s? t:f=w156:T13)
      }
      frame "Init Auto SPI" {
        w167 = u8 26 ("dimension size")
        # "An extra two bytes are needed to complete the read. NULL bytes were added because the AutoSPI controller \nonly supports byte (8-bit) transactions. The IMU requires two bytes (16-bits) per CS."
        n59 = Unbundle By Name(w178) -> ("ADIS16448DevRef.Hardware Config.Stall Config"=w177:T21, "Digital Source"=w175:T8, "SPIDevRef.SPI Bus"=w174:T6)
        n60 = Build Array(u8 62 ("hi"), u8 0 ("element")) -> (w168:u8[])
        n61 = Array Size(array=w168) -> (size(s)=w172:i32)
        n62 = Add(x=w172, y=w167) -> (x+y=w169:i32)
        n63 = call <vilib>:"FPGA_SPI_ConfigureAuto.vi"("SPI Auto Zero Byte Count"=w167, "error in"=w182, "SPI Auto TX Byte Array"=w168, "Stall Config"=w177, "SPI Bus"=w174) -> ("error out"=w181:errorcluster)  [unwired: 6 in]
        n64 = call <vilib>:"FPGA_SPI_StartAuto_External.vi"("error in (no error)"=w181, "Falling Edge"=FALSE, "Rising Edge"=TRUE, "Source"=w175) -> ("error out"=w166:errorcluster)  [unwired: 7 in]
        n65 = Bundle By Name(cluster=w178, "Bytes Per Sample"=w169, "AutoSPI Active?"=TRUE, "Reset"=TRUE, "Data Header"=w168, "Zero Byte Count"=w167) -> (w164:T14)
      }
      frame "***Calibration***" {
        # "#NOTE JAS should never\nget to this state"
      }
      frame "Calibrate" {
        n66 = Unbundle By Name(w191) -> ("AutoSPI Active?"=w198:bool, "Bytes Per Sample"=w195:u32, "Offset Counter"=w194:i32, "ADIS16448DevRef.Calibration Time"=w193:u32)
        n67 = case shown="True" w198 {
          tunnel: [w201 w219] -> w188
          tunnel: w197 -> [w200 w214]
          tunnel: [w200 w205] -> w196
          tunnel: w191 -> [w201 w215]
          tunnel: w195 -> [_ w212]
          tunnel: w194 -> [_ w209]
          tunnel: w193 -> [_ w210]
          tunnel: [ADIS16448_Loop_State."Reset" w206] -> w192
          frame False {
          }
          frame True {
            n68 = Multiply(x=819, y=w210) -> (x*y=w203:u32)
            n69 = call <vilib>:"FPGA_SPI_ReadAuto.vi"("error in (no error)"=w214, "Bytes per Sample"=w212, "Samples to Read"=u32 0) -> ("error out"=w213:errorcluster, "Timestamps"=w216:u32[], "Data"=w217:u8[][])  [unwired: 6 in]
            n70 = for {
              tunnel: w217 -> [w237] mode=indexing
              tunnel: w216 -> [_] mode=indexing
              tunnel: w213 -> [w236]
              tunnel: [w233] -> w204
              shift-right: [w234] -> w202
              shift-left: w209 -> [w227]
              tunnel: w203 -> [w231]
              # "Throw away first n samples"
              n71 = call "ADIS16448 Scale Data.vi"("error in (no error)"=w236, "New Data In"=w237) -> ("error out"=w232:errorcluster, "Data Good?"=w229:bool, "Data Out"=w235:dbl[])  [unwired: 7 in]
              n72 = Greater?(x=w227, y=10.0) -> (0:w226:bool)
              n73 = And(x=w226, y=w229) -> (x .and. y?=w228:bool)
              n74 = case shown="True" w228 {
                tunnel: w235 -> [_ w245]
                tunnel: w227 -> [w239 w243]
                tunnel: [w238 w242] -> w234
                tunnel: [w240 w244] -> w233
                tunnel: w232 -> [w240 w244]
                tunnel: w231 -> [_ w241]
                frame False {
                  n75 = Increment(x=w239) -> (x+1=w238:i32)
                }
                frame True {
                  n76 = Increment(x=w243) -> (x+1=w242:i32)
                  n77 = call "ADIS16448 Loop Manage Cal Buffer.vi"("Sample Count"=w241, "Data In"=w245) -> ()  [unwired: 9 in, 1 out]
                }
              }
            }
            n78 = Greater?(x=w202, y=w203) -> (0:w208:bool)
            n79 = case shown="True" w208 {
              tunnel: w202 -> [w222 _]
              tunnel: [w222 u32 0 ("Offset Counter")] -> w207
              tunnel: [ADIS16448_Loop_State."Calibrate" ADIS16448_Loop_State."Finish Cal"] -> w206
              tunnel: [w220 w223] -> w205
              tunnel: w204 -> [w220 w223]
              frame False {
              }
              frame True {
              }
            }
            n80 = global write "ADIS16448 Globals.vi" "Calibration Count"(w202) -> ()
            n81 = Bundle By Name(cluster=w215, "Offset Counter"=w207) -> (w219:T14)
          }
        }
        n82 = Wait (ms)(milliseconds to wait=u32 20) -> ()  [unwired: 1 out]
      }
      frame "Finish Cal" {
        # "#NOTE Was RUN"
        # "Drive MXP PWM5 (IMU \nready LED) low (active low)"
        n83 = disable-structure shown="Disabled" {
          disable-tunnel: w257 -> [w271 _]
          disable-tunnel: w256 -> [w270 _]
          disable-tunnel: [w263 _] -> w255
          frame Disabled {
            n84 = Unbundle By Name(w270) -> ("ADIS16448DevRef.Calibration Complete"=w273:refnum<notifier>)
            n85 = Unbundle By Name(w270) -> ("ADIS16448DevRef.Hardware Config.IMU Status LED Pin"=w261:T5)
            n86 = Send Notification(notification="", notifier=w273, error in (no error)=w271) -> (error out=w264:errorcluster)  [unwired: 1 out]
            n87 = call <vilib>:"WPI_DigitalOutputOpen.vi"("error in (no error)"=w264, "DIO Channel"=w261) -> ("error out"=w269:errorcluster, "DigitalOutputDevRef"=w268:T19)  [unwired: 8 in]
            n88 = call <vilib>:"WPI_DigitalOutputSetValue.vi"("error in (no error)"=w269, "Value"=FALSE, "DigitalOutputDevRef"=w268) -> ("error out"=w267:errorcluster, "DigitalOutputDevRef"=w266:T19)  [unwired: 7 in]
            n89 = call <vilib>:"WPI_DigitalOutputRefNum Registry Set.vi"("error in (no error)"=w267, "refnum name"="448 Status LED", "DigitalOutputDevRef"=w266) -> ("error out"=w263:errorcluster)  [unwired: 7 in, 1 out]
          }
          frame Enabled {
          }
        }
        n90 = call "ADIS16448 Loop Update Status.vi"("ADIS16448 Status"=T16 {"Calibrated?"=TRUE, "IMU Detected?"=TRUE} ("element")) -> ()  [unwired: 10 in, 1 out]
        n91 = case shown="True" w250 {
          frame False {
            n92 = call <vilib>:"WPI_UtilitiesFRC SendMessageToConsole.vi"("Message"="ADIS16448 IMU Successfully Initialized!" ("format string")) -> ()  [unwired: 14 in, 1 out]
          }
          frame True {
            n93 = call <vilib>:"WPI_UtilitiesFRC SendMessageToConsole.vi"("Message"="ADIS16448 IMU Successfully Initialized!   Using register read mode" ("format string")) -> ()  [unwired: 14 in, 1 out]
          }
        }
        n94 = call "ADIS16448 Loop Manage Cal Buffer.vi"("Cmd"=ADIS16448_Call_Buffer_Cmd."Calculate") -> ("Cal Offset Out"=w247:dbl[])  [unwired: 10 in]
        n95 = Bundle By Name(cluster=w256, "Reset"=TRUE ("First Run"), "Offsets"=w247) -> (w246:T14)
        n96 = Select(t=ADIS16448_Loop_State."Run_Alt", s=w250, f=ADIS16448_Loop_State."Run") -> (s? t:f=w252:T13)
      }
      frame "***Operation***" {
        # "#NOTE JAS should never get to this state"
      }
      frame "Run" {
        # "#NOTE The data calcuation is only correct for gyro readings..."
        # "#NOTE\nJAS moved \nwait to get data to users\nfaster."
        # "Main data capture and accumulation loop. Only active if AutoSPI is enabled."
        n97 = Unbundle By Name(w281) -> ("AutoSPI Active?"=w280:bool)
        n98 = case shown="True" w280 {
          tunnel: [w286 w306] -> w278
          tunnel: w283 -> [w285 w299]
          tunnel: [w285 w297] -> w282
          tunnel: w281 -> [w286 w292]
          tunnel: w281 -> [_ w293]
          frame False {
          }
          frame True {
            # "#NOTE Use my post scale routine.  It might benefit\nfrom some performance enhancements."
            n99 = Unbundle By Name(w293) -> ("Data"=w290:dbl[], "Offsets"=w289:dbl[], "Reset"=w288:bool, "Bytes Per Sample"=w305:u32)
            n100 = Unbundle By Name(w293) -> ("ADIS16448DevRef.Calibration Time"=w295:u32, "TimeStampPrev"=w301:u32)
            n101 = call <vilib>:"FPGA_SPI_ReadAuto.vi"("error in (no error)"=w299, "Bytes per Sample"=w305, "Samples to Read"=u32 0) -> ("error out"=w298:errorcluster, "Timestamps"=w302:u32[], "Data"=w303:u8[][])  [unwired: 6 in]
            n102 = Multiply(x=819, y=w295) -> (x*y=w294:u32)
            n103 = for {
              tunnel: w303 -> [w323] mode=indexing
              tunnel: w302 -> [w314] mode=indexing
              shift-right: [w314] -> w300
              shift-left: w301 -> [w324]
              tunnel: w298 -> [w322]
              tunnel: [w312] -> w297
              tunnel: w294 -> [w313]
              shift-right: [w310] -> w291
              shift-left: w290 -> [w311]
              tunnel: w289 -> [w309]
              tunnel: w288 -> [w308]
              tunnel: [w307] -> w287
              n104 = Subtract(x=w314, y=w324) -> (x-y=w321:u32)
              n105 = call "ADIS16448 Scale Data.vi"("error in (no error)"=w322, "New Data In"=w323) -> ("error out"=w312:errorcluster, "Data Good?"=w317:bool, "Data Out"=w315:dbl[])  [unwired: 7 in]
              n106 = Divide(x=w321, y=u32 1000000) -> (x/y=w319:dbl)
              n107 = First Call?() -> (First Call?: T/F=w316:bool)
              n108 = Or(x=w316, y=w317) -> (x .or. y?=w318:bool)
              n109 = case shown="True" w318 {
                tunnel: w315 -> [_ w331]
                tunnel: w319 -> [_ w333]
                tunnel: [w326 w334] -> w310
                tunnel: w313 -> [_ w332]
                tunnel: w311 -> [w326 w330]
                tunnel: w309 -> [_ w329]
                tunnel: w308 -> [w325 w328]
                tunnel: [w325 w327] -> w307
                frame False {
                }
                frame True {
                  n110 = call "ADIS16448 Loop Manage Cal Buffer.vi"("Sample Count"=w332, "Data In"=w331) -> ()  [unwired: 9 in, 1 out]
                  n111 = call "ADIS16448 Loop Post Scale.vi"("TimePeriod"=w333, "Reset"=w328, "Data In"=w330, "Offsets"=w329, "Scaled Data In"=w331) -> ("Reset Out"=w327:bool, "Data Out"=w334:dbl[])  [unwired: 5 in]
                }
              }
            }
            n112 = call "ADIS16448 Loop Inc Acquire Count.vi"() -> ()  [unwired: 11 in, 1 out]
            n113 = Bundle By Name(cluster=w292, "Data"=w291, "Reset"=w287, "TimeStampPrev"=w300) -> (w306:T14)
          }
        }
      }
      frame "Process" {
        # "#NOTE Run faster in register mode since no auto queue of data"
        # "#NOTE The other data is missing from"
        n114 = Unbundle By Name(w335) -> ("ADIS16448DevRef.Sychronous Process VI"=w343:T7, "Data"=w336:dbl[])
        n115 = Not A Number/Path/Refnum?(number/path/refnum=w343) -> (NaN/Path/Refnum?=w344:bool)
        n116 = case shown="False" w344 {
          tunnel: w346 -> [w354 w359]
          tunnel: [w358 w359] -> w345
          tunnel: w343 -> [w357 _]
          tunnel: w336 -> [w352 _]
          frame False {
            n117 = Index Array(array=w352) -> (element #1=w351:dbl, element #2=w350:dbl, element #3=w349:dbl)  [unwired: 3 in]
            n118 = Bundle By Name(cluster="element", "XAngle"=w351, "YAngle"=w350, "ZAngle"=w349) -> ()  [unwired: 1 out]
            n119 = call-by-ref "?"(reference=w357, error in=w354, 8:"error in (no error)"=w354) -> (error out=w355:errorcluster, 0:"error out"=w356:errorcluster)  [unwired: 10 in, 1 out]
            n120 = Merge Errors(w355, w356) -> (w358:errorcluster)
          }
          frame True {
          }
        }
        n121 = case shown="True" w338 {
          tunnel: [u32 20 ("milliseconds to wait") u32 10 ("milliseconds to wait")] -> w337
          frame False {
          }
          frame True {
          }
        }
        n122 = Wait (ms)(milliseconds to wait=w337) -> ()  [unwired: 1 out]
        n123 = Select(t=ADIS16448_Loop_State."Run_Cmds_Alt", s=w338, f=ADIS16448_Loop_State."Run Cmds") -> (s? t:f=w340:T13)
      }
      frame "Run Cmds" {
        n124 = Unbundle By Name(w364) -> ("ADIS16448DevRef.Cmd FIFO"=w371:refnum<k33>)
        n125 = Unbundle By Name(w364) -> ("ADIS16448DevRef.Calibration Complete"=w368:refnum<notifier>)
        n126 = RT FIFO Read(0:w371, 1:T18 {"Command"=enum."None", "Data"=0} ("element")) -> (8:w367:refnum<k33>, 9:w366:T18)  [unwired: 2 in, 3 out]
        n127 = Unbundle(w366) -> ("Command"=w363:T22, "Data"=w365:u32)
        n128 = case shown="\"Recalibrate\"" w363 {
          tunnel: w364 -> [w374 w380 w384 w395 w404 w418 w463 w481 w486]
          tunnel: w370 -> [w375 w379 w386 w393 w407 w434 w473 w482 w487]
          tunnel: [w375 w379 w381 w393 w407 w421 w464 w482 w487] -> w369
          tunnel: [w374 w378 w383 w396 w403 w417 w463 w481 w485] -> w360
          tunnel: w368 -> [_ _ _ _ w406 _ _ _ _]
          tunnel: w367 -> [_ _ w389 w398 _ w432 w475 w478 _]
          tunnel: w365 -> [_ _ _ _ _ _ _ _ w483]
          tunnel: w364 -> [_ _ w385 _ _ w415 w462 _ _]
          tunnel: [ADIS16448_Loop_State."Run" ADIS16448_Loop_State."Run" ADIS16448_Loop_State."Run" ADIS16448_Loop_State."Run" ADIS16448_Loop_State."Run" w409 ADIS16448_Loop_State."Run" ADIS16448_Loop_State."Run" ADIS16448_Loop_State."Run"] -> w362
          frame "None", Default {
          }
          frame "Reset" {
            n129 = Bundle By Name(cluster=w380, "Reset"=TRUE ("First Run")) -> (w378:T14)
          }
          frame "Rewrite Config" {
            # "#NOTE JAS replaced with func"
            n130 = Unbundle By Name(w385) -> ("SPIDevRef"=w387:T15)
            n131 = RT FIFO Write(0:w389, 1:T18 {"Command"=enum."Start Auto SPI", "Data"=0} ("element")) -> ()  [unwired: 3 in, 4 out]
            n132 = call "ADIS16448 Loop Write Config.vi"("error in (no error)"=w386, "SPIDevRef"=w387) -> ("error out"=w381:errorcluster, "SPIDevRef out"=w382:T15)  [unwired: 8 in]
            n133 = Bundle By Name(cluster=w384, "SPIDevRef"=w382) -> (w383:T14)
          }
          frame "Recalibrate" {
            n134 = RT FIFO Write(0:w398, 1:T18 {"Command"=enum."Recal Complete", "Data"=0} ("element")) -> ()  [unwired: 3 in, 4 out]
            n135 = call "ADIS16448 Loop Manage Cal Buffer.vi"("Cmd"=ADIS16448_Call_Buffer_Cmd."Calculate") -> ("Cal Offset Out"=w391:dbl[])  [unwired: 10 in]
            n136 = global write "ADIS16448 Globals.vi" "CallOffsets"(w391) -> ()
            n137 = Bundle By Name(cluster=w395, "Offsets"=w391) -> (w396:T14)
          }
          frame "Recal Complete" {
            n138 = call "ADIS16448 Loop Update Status.vi"("ADIS16448 Status"=T16 {"Calibrated?"=TRUE, "IMU Detected?"=TRUE} ("element")) -> ()  [unwired: 10 in, 1 out]
            n139 = Send Notification(notification="", notifier=w406) -> ()  [unwired: 1 in, 2 out]
            n140 = Bundle By Name(cluster=w404, "AutoSPI Active?"=TRUE, "Reset"=TRUE) -> (w403:T14)
          }
          frame "Exit Auto SPI" {
            w428 = T12 114 items=["Reserved1"=0, "DIAG_STAT"=2, "X_GYRO_LOW"=4, "X_GYRO_OUT"=6, "Y_GYRO_LOW"=8, "Y_GYRO_OUT"=10, "Z_GYRO_LOW"=12, "Z_GYRO_OUT"=14, "X_ACCL_LOW"=16, "X_ACCL_OUT"=18, "Y_ACCL_LOW"=20, "Y_ACCL_OUT"=22, "Z_ACCL_LOW"=24, "Z_ACCL_OUT"=26, "TEMP_OUT"=28, "TIME_STAMP"=30, "Reseved2"=32, "DATA_CNTR"=34, "X_DELTANG_LOW"=36, "X_DELTANG_OUT"=38, "Y_DELTANG_LOW"=40, "Y_DELTANG_OUT"=42, "Z_DELTANG_LOW"=44, "Z_DELTANG_OUT"=46, "X_DELTVEL_LOW"=48, "X_DELTVEL_OUT"=50, "Y_DELTVEL_LOW"=52, "Y_DELTVEL_OUT"=54, "Z_DELTVEL_LOW"=56, "Z_DELTVEL_OUT"=58, "Reserved3"=60, "Reserved4"=62, "XG_BIAS_LOW"=64, "XG_BIAS_HIGH"=66, "YG_BIAS_LOW"=68, "YG_BIAS_OUT"=70, "ZG_BIAS_LOW"=72, "ZG_BIAS_OUT"=74, "XA_BIAS_LOW"=76, "XA_BIAS_HIGH"=78, "YA_BIAS_LOW"=80, "YA_BIAS_OUT"=82, "ZA_BIAS_LOW"=84, "ZA_BIAS_OUT"=86, "Reserved5"=88, "Reserved6"=90, "FILT_CTRL"=92, "Reserved5"=94, "MSC_CTRL"=96, "UP_SCALE"=98, "DEC_RATE"=100, "NULL_CNFG"=102, "GLOB_CMD"=104, "Reserved6"=106, "FIRM_REV"=108, "FIRM_DM"=110, "FIRM_Y"=112, "PROD_ID"=114, "SERIAL_NUM"=116, "USER_SCR1"=118, "USER_SCR2"=120, "USER_SCR3"=122, "FLSHCNT_LOW"=124, "FLSHCNT_HIGH"=126] ("ADIS16448 Register")
            # "#TODO Should be function"
            n141 = Unbundle By Name(w415) -> ("ADIS16448DevRef.Hardware Config.IMU SPI Bus"=w431:T6, "ADIS16448DevRef.Hardware Config.SPI Clock Rate (Hz)"=w430:dbl, "ADIS16448DevRef.Hardware Config.IMU SPI Mode (3)"=w429:T4, "SPIDevRef"=w410:T15)
            n142 = call "ADIS16448 Loop Update Status.vi"("ADIS16448 Status"=T16 {"Calibrated?"=FALSE, "IMU Detected?"=FALSE} ("element")) -> ()  [unwired: 10 in, 1 out]
            n143 = RT FIFO Write(0:w432, 1:T18 {"Command"=enum."Rewrite Config", "Data"=0} ("element")) -> ()  [unwired: 3 in, 4 out]
            n144 = call <vilib>:"WPI_SPIClose.vi"("error in (no error)"=w434, "SPIDevRef"=w410) -> ("error out"=w419:errorcluster)  [unwired: 9 in]
            n145 = call <vilib>:"WPI_DigitalOutputRefNum Registry Get.vi"("error in (no error)"=w419, "refnum name"="448 Status LED") -> ("error out"=w413:errorcluster, "DigitalOutputDevRef"=w412:T19)  [unwired: 8 in]
            n146 = call <vilib>:"WPI_DigitalOutputSetValue.vi"("error in (no error)"=w413, "Value"=TRUE, "DigitalOutputDevRef"=w412) -> ("error out"=w414:errorcluster)  [unwired: 7 in, 1 out]
            n147 = call <vilib>:"WPI_SPIOpen.vi"("error in"=w414, "Mode (3)"=w429, "Clock Rate (Hz)"=w430, "SPI Bus"=w431) -> ("error out"=w427:errorcluster, "SPIDevRef"=w423:T15)  [unwired: 6 in]
            n148 = call "ADIS16448 Read Register.vi"("error in (no error)"=w427, "ADIS16448 Register"=w428, "SPIDevRef in"=w423) -> ("error out"=w424:errorcluster, "Register Value"=w422:u16, "SPIDevRef out"=w425:T15)  [unwired: 6 in]
            n149 = Equal?(x=u16 16448 ("y"), y=w422) -> (x = y?=w426:bool)
            n150 = case shown="True" w426 {
              tunnel: w425 -> [w437 w453]
              tunnel: w424 -> [w438 w452]
              tunnel: [w440 w451] -> w421
              tunnel: w418 -> [w439 w449]
              tunnel: [w439 w448] -> w417
              tunnel: [ADIS16448_Loop_State."Reset" ADIS16448_Loop_State."Run"] -> w409
              frame False {
                n151 = call <vilib>:"WPI_SPIClose.vi"("error in (no error)"=w438, "SPIDevRef"=w437) -> ("error out"=w436:errorcluster)  [unwired: 9 in]
                n152 = case shown="No Error" w436 {
                  selector: w436 -> [w442 w445]
                  tunnel: [w441 w445] -> w440
                  frame No Error {
                    n153 = call <vilib>:"Error Cluster From Error Code.vi"("error in (no error)"=w442, "error message (\"\")"="SPI port did not reset properly" ("error message (\"\")"), "error code (0)"=-8106) -> ("error out"=w441:errorcluster)  [unwired: 6 in]
                  }
                  frame Error {
                  }
                }
              }
              frame True {
                n154 = call <vilib>:"WPI_SPIRefNum Registry Set.vi"("error in (no error)"=w452, "refnum name"="AutoSPI", "SPIDevRef"=w453) -> ("error out"=w451:errorcluster, "SPIDevRef"=w454:T15)  [unwired: 7 in]
                n155 = call "ADIS16448 Loop Update Status.vi"("ADIS16448 Status"=T16 {"Calibrated?"=FALSE, "IMU Detected?"=TRUE} ("element")) -> ()  [unwired: 10 in, 1 out]
                n156 = Bundle By Name(cluster=w449, "SPIDevRef"=w454, "AutoSPI Active?"=FALSE) -> (w448:T14)
              }
            }
          }
          frame "Start Auto SPI" {
            # "#TODO Should be function"
            n157 = Unbundle By Name(w462) -> ("SPIDevRef"=w461:T15, "Digital Source"=w460:T8, "ADIS16448DevRef.Hardware Config.Stall Config"=w459:T21, "Data Header"=w458:u8[], "Zero Byte Count"=w457:u8)
            n158 = Unbundle By Name(w461) -> ("SPI Bus"=w474:T6)
            n159 = RT FIFO Write(0:w475, 1:T18 {"Command"=enum."Recal Complete", "Data"=0} ("element")) -> ()  [unwired: 3 in, 4 out]
            n160 = call <vilib>:"FPGA_SPI_ConfigureAuto.vi"("SPI Auto Zero Byte Count"=w457, "error in"=w473, "SPI Auto TX Byte Array"=w458, "Stall Config"=w459, "SPI Bus"=w474) -> ("error out"=w466:errorcluster)  [unwired: 6 in]
            n161 = call <vilib>:"FPGA_SPI_StartAuto_External.vi"("error in (no error)"=w466, "Falling Edge"=FALSE, "Rising Edge"=TRUE, "Source"=w460) -> ("error out"=w470:errorcluster)  [unwired: 7 in]
            n162 = call <vilib>:"WPI_DigitalOutputRefNum Registry Get.vi"("error in (no error)"=w470, "refnum name"="448 Status LED") -> ("error out"=w469:errorcluster, "DigitalOutputDevRef"=w468:T19)  [unwired: 8 in]
            n163 = call <vilib>:"WPI_DigitalOutputSetValue.vi"("error in (no error)"=w469, "Value"=FALSE, "DigitalOutputDevRef"=w468) -> ("error out"=w464:errorcluster)  [unwired: 7 in, 1 out]
          }
          frame "Start Recal" {
            n164 = call "ADIS16448 Loop Update Status.vi"("ADIS16448 Status"=T16 {"Calibrated?"=FALSE, "IMU Detected?"=TRUE} ("element")) -> ()  [unwired: 10 in, 1 out]
            n165 = RT FIFO Write(0:w478, 1:T18 {"Command"=enum."Recalibrate", "Data"=0} ("element")) -> ()  [unwired: 3 in, 4 out]
          }
          frame "Configure Cal" {
            n166 = Bundle By Name(cluster=w486, "ADIS16448DevRef.Calibration Time"=w483) -> (w485:T14)
          }
        }
      }
      frame "Run_Alt" {
        n167 = in-place {
          in-place-border: w495 -> [w512]
          in-place-border: [w498] -> w493
          in-place-border: w492 -> [w508]
          in-place-border: [w507] -> w491
          in-place-border: w490 -> [w506]
          in-place-border: w489 -> [w505]
          # "read registers one at a time...."
          n168 = in-place-cluster #1(w489) -> ("Data"=w500:dbl[], "Reset"=w499:bool)
          n169 = Unbundle By Name(w505) -> ("SPIDevRef"=w513:T15, "CalSamplesAlt"=w503:i32, "Offsets"=w501:dbl[])
          n170 = for {
            tunnel: w506 -> [w526] mode=indexing
            shift-right: [w519] -> w511
            shift-left: w512 -> [w523]
            shift-right: [w514] -> _
            shift-left: w513 -> [w525]
            shift-right: [w515] -> w507
            shift-left: w508 -> [w522]
            # "hi\nlow"
            n171 = Unbundle(w526) -> ("Reg"=w524:T12, "Data"=w521:u16)
            n172 = call "ADIS16448 Read Register.vi"("error in (no error)"=w523, "ADIS16448 Register"=w524, "SPIDevRef in"=w525) -> ("error out"=w519:errorcluster, "Register Value"=w518:u16, "SPIDevRef out"=w514:T15)  [unwired: 6 in]
            n173 = Increment(x=w521) -> (x+1=w520:u16)
            n174 = Split Number(x=w518) -> (hi(x)=w517:u8, lo(x)=w516:u8)
            n175 = Replace Array Subset(array=w522, new element #1=w517, index #1=w521, new element #2=w516, index #2=w520) -> (w515:u8[])
          }
          n176 = call "ADIS16448 Scale Data_Alt.vi"("error in (no error)"=w511, "New Data In"=w507) -> ("error out"=w498:errorcluster, "Data Out"=w502:dbl[])  [unwired: 7 in, 1 out]
          n177 = call "ADIS16448 Loop Manage Cal Buffer.vi"("Sample Count"=w503, "Data In"=w502) -> ()  [unwired: 9 in, 1 out]
          n178 = call "ADIS16448 Loop Inc Acquire Count.vi"() -> ()  [unwired: 11 in, 1 out]
          n179 = call <vilib>:"Util_GetTime.vi"() -> ("FPGA_Time_Seconds"=w510:dbl)  [unwired: 10 in, 1 out]
          n180 = feedback #2(w510) -> (w509:dbl)
          n181 = feedback-in #2(w510) -> ()
          n182 = Subtract(x=w510, y=w509) -> (x-y=w504:dbl)
          n183 = call "ADIS16448 Loop Post Scale.vi"("TimePeriod"=w504, "Reset"=w499, "Data In"=w500, "Offsets"=w501, "Scaled Data In"=w502) -> ("Reset Out"=w496:bool, "Data Out"=w497:dbl[])  [unwired: 5 in]
          n184 = in-place-cluster #1("Data"=w497, "Reset"=w496) -> (w488:T14)
        }
      }
      frame "Run_Cmds_Alt" {
        n185 = Unbundle By Name(w530) -> ("ADIS16448DevRef.Cmd FIFO"=w537:refnum<k33>)
        n186 = Unbundle By Name(w530) -> ("ADIS16448DevRef.Calibration Complete"=w536:refnum<notifier>)
        n187 = RT FIFO Read(0:w537, 1:T18 {"Command"=enum."None", "Data"=0} ("element")) -> (8:w535:refnum<k33>, 9:w534:T18)  [unwired: 2 in, 3 out]
        n188 = Unbundle(w534) -> ("Command"=w532:T22, "Data"=w533:u32)
        n189 = case shown="\"Recalibrate\"" w532 {
          tunnel: w530 -> [w541 w547 w555 w565 w575 w591 w632 w658 w666]
          tunnel: w531 -> [w542 w546 w551 w563 w578 w607 w634 w659 w667]
          tunnel: [w542 w546 w550 w563 w578 w594 w633 w659 w667] -> w529
          tunnel: [w541 w545 w554 w566 w574 w590 w632 w658 w665] -> w527
          tunnel: w536 -> [_ _ _ _ w577 _ _ _ _]
          tunnel: w535 -> [_ _ w558 w568 _ w605 w635 w655 _]
          tunnel: w533 -> [_ _ _ _ _ _ _ _ w661]
          tunnel: w530 -> [_ _ w557 _ _ w588 w631 _ _]
          tunnel: [ADIS16448_Loop_State."Run_Alt" ADIS16448_Loop_State."Run_Alt" ADIS16448_Loop_State."Run_Alt" ADIS16448_Loop_State."Run_Alt" ADIS16448_Loop_State."Run_Alt" w582 ADIS16448_Loop_State."Run_Alt" ADIS16448_Loop_State."Run_Alt" ADIS16448_Loop_State."Run_Alt"] -> w528
          frame "None", Default {
          }
          frame "Reset" {
            n190 = disable-structure shown="Disabled" {
              frame Disabled {
                n191 = call <vilib>:"WPI_UtilitiesFRC SendMessageToConsole.vi"("Message"="ADIS16448 Alt Reset requested" ("format string")) -> ()  [unwired: 14 in, 1 out]
              }
              frame Enabled {
              }
            }
            n192 = Bundle By Name(cluster=w547, "Reset"=TRUE ("First Run")) -> (w545:T14)
          }
          frame "Rewrite Config" {
            # "#NOTE Shouldn't do this in register mode...."
            n193 = disable-structure shown="Disabled" {
              disable-tunnel: w558 -> [w559 _]
              frame Disabled {
                n194 = RT FIFO Write(0:w559, 1:T18 {"Command"=enum."Start Auto SPI", "Data"=0} ("element")) -> ()  [unwired: 3 in, 4 out]
              }
              frame Enabled {
              }
            }
            n195 = Unbundle By Name(w557) -> ("SPIDevRef"=w552:T15)
            n196 = call <vilib>:"WPI_UtilitiesFRC SendMessageToConsole.vi"("Message"="ADIS16448 Alt write config requested" ("format string")) -> ()  [unwired: 14 in, 1 out]
            n197 = call "ADIS16448 Loop Write Config.vi"("error in (no error)"=w551, "SPIDevRef"=w552) -> ("error out"=w550:errorcluster, "SPIDevRef out"=w553:T15)  [unwired: 8 in]
            n198 = Bundle By Name(cluster=w555, "SPIDevRef"=w553) -> (w554:T14)
          }
          frame "Recalibrate" {
            n199 = disable-structure shown="Disabled" {
              frame Disabled {
                n200 = call <vilib>:"WPI_UtilitiesFRC SendMessageToConsole.vi"("Message"="ADIS16448 Alt recalibrate requested" ("format string")) -> ()  [unwired: 14 in, 1 out]
              }
              frame Enabled {
              }
            }
            n201 = RT FIFO Write(0:w568, 1:T18 {"Command"=enum."Recal Complete", "Data"=0} ("element")) -> ()  [unwired: 3 in, 4 out]
            n202 = call "ADIS16448 Loop Manage Cal Buffer.vi"("Cmd"=ADIS16448_Call_Buffer_Cmd."Calculate") -> ("Cal Offset Out"=w561:dbl[])  [unwired: 10 in]
            n203 = global write "ADIS16448 Globals.vi" "CallOffsets"(w561) -> ()
            n204 = Bundle By Name(cluster=w565, "Offsets"=w561) -> (w566:T14)
          }
          frame "Recal Complete" {
            n205 = Send Notification(notification="", notifier=w577) -> ()  [unwired: 1 in, 2 out]
            n206 = call "ADIS16448 Loop Update Status.vi"("ADIS16448 Status"=T16 {"Calibrated?"=TRUE, "IMU Detected?"=TRUE} ("element")) -> ()  [unwired: 10 in, 1 out]
            n207 = disable-structure shown="Disabled" {
              frame Disabled {
                n208 = call <vilib>:"WPI_UtilitiesFRC SendMessageToConsole.vi"("Message"="ADIS16448 Alt recal complete" ("format string")) -> ()  [unwired: 14 in, 1 out]
              }
              frame Enabled {
              }
            }
            n209 = Bundle By Name(cluster=w575, "AutoSPI Active?"=TRUE, "Reset"=TRUE) -> (w574:T14)
          }
          frame "Exit Auto SPI" {
            w601 = T12 114 items=["Reserved1"=0, "DIAG_STAT"=2, "X_GYRO_LOW"=4, "X_GYRO_OUT"=6, "Y_GYRO_LOW"=8, "Y_GYRO_OUT"=10, "Z_GYRO_LOW"=12, "Z_GYRO_OUT"=14, "X_ACCL_LOW"=16, "X_ACCL_OUT"=18, "Y_ACCL_LOW"=20, "Y_ACCL_OUT"=22, "Z_ACCL_LOW"=24, "Z_ACCL_OUT"=26, "TEMP_OUT"=28, "TIME_STAMP"=30, "Reseved2"=32, "DATA_CNTR"=34, "X_DELTANG_LOW"=36, "X_DELTANG_OUT"=38, "Y_DELTANG_LOW"=40, "Y_DELTANG_OUT"=42, "Z_DELTANG_LOW"=44, "Z_DELTANG_OUT"=46, "X_DELTVEL_LOW"=48, "X_DELTVEL_OUT"=50, "Y_DELTVEL_LOW"=52, "Y_DELTVEL_OUT"=54, "Z_DELTVEL_LOW"=56, "Z_DELTVEL_OUT"=58, "Reserved3"=60, "Reserved4"=62, "XG_BIAS_LOW"=64, "XG_BIAS_HIGH"=66, "YG_BIAS_LOW"=68, "YG_BIAS_OUT"=70, "ZG_BIAS_LOW"=72, "ZG_BIAS_OUT"=74, "XA_BIAS_LOW"=76, "XA_BIAS_HIGH"=78, "YA_BIAS_LOW"=80, "YA_BIAS_OUT"=82, "ZA_BIAS_LOW"=84, "ZA_BIAS_OUT"=86, "Reserved5"=88, "Reserved6"=90, "FILT_CTRL"=92, "Reserved5"=94, "MSC_CTRL"=96, "UP_SCALE"=98, "DEC_RATE"=100, "NULL_CNFG"=102, "GLOB_CMD"=104, "Reserved6"=106, "FIRM_REV"=108, "FIRM_DM"=110, "FIRM_Y"=112, "PROD_ID"=114, "SERIAL_NUM"=116, "USER_SCR1"=118, "USER_SCR2"=120, "USER_SCR3"=122, "FLSHCNT_LOW"=124, "FLSHCNT_HIGH"=126] ("ADIS16448 Register")
            n210 = Unbundle By Name(w588) -> ("ADIS16448DevRef.Hardware Config.IMU SPI Bus"=w604:T6, "ADIS16448DevRef.Hardware Config.SPI Clock Rate (Hz)"=w603:dbl, "ADIS16448DevRef.Hardware Config.IMU SPI Mode (3)"=w602:T4, "SPIDevRef"=w583:T15)
            n211 = call "ADIS16448 Loop Update Status.vi"("ADIS16448 Status"=T16 {"Calibrated?"=FALSE, "IMU Detected?"=FALSE} ("element")) -> ()  [unwired: 10 in, 1 out]
            n212 = RT FIFO Write(0:w605, 1:T18 {"Command"=enum."Rewrite Config", "Data"=0} ("element")) -> ()  [unwired: 3 in, 4 out]
            n213 = call <vilib>:"WPI_SPIClose.vi"("error in (no error)"=w607, "SPIDevRef"=w583) -> ("error out"=w592:errorcluster)  [unwired: 9 in]
            n214 = call <vilib>:"WPI_DigitalOutputRefNum Registry Get.vi"("error in (no error)"=w592, "refnum name"="448 Status LED") -> ("error out"=w586:errorcluster, "DigitalOutputDevRef"=w585:T19)  [unwired: 8 in]
            n215 = call <vilib>:"WPI_DigitalOutputSetValue.vi"("error in (no error)"=w586, "Value"=TRUE, "DigitalOutputDevRef"=w585) -> ("error out"=w587:errorcluster)  [unwired: 7 in, 1 out]
            n216 = call <vilib>:"WPI_SPIOpen.vi"("error in"=w587, "Mode (3)"=w602, "Clock Rate (Hz)"=w603, "SPI Bus"=w604) -> ("error out"=w600:errorcluster, "SPIDevRef"=w596:T15)  [unwired: 6 in]
            n217 = call <vilib>:"WPI_UtilitiesFRC SendMessageToConsole.vi"("Message"="ADIS16448 Alt exit auto SPI requested" ("format string")) -> ()  [unwired: 14 in, 1 out]
            n218 = call "ADIS16448 Read Register.vi"("error in (no error)"=w600, "ADIS16448 Register"=w601, "SPIDevRef in"=w596) -> ("error out"=w597:errorcluster, "Register Value"=w595:u16, "SPIDevRef out"=w598:T15)  [unwired: 6 in]
            n219 = Equal?(x=u16 16448 ("y"), y=w595) -> (x = y?=w599:bool)
            n220 = case shown="True" w599 {
              tunnel: w598 -> [w610 w626]
              tunnel: w597 -> [w611 w625]
              tunnel: [w613 w624] -> w594
              tunnel: w591 -> [w612 w622]
              tunnel: [w612 w621] -> w590
              tunnel: [ADIS16448_Loop_State."Reset" ADIS16448_Loop_State."Run_Alt"] -> w582
              frame False {
                n221 = call <vilib>:"WPI_SPIClose.vi"("error in (no error)"=w611, "SPIDevRef"=w610) -> ("error out"=w609:errorcluster)  [unwired: 9 in]
                n222 = case shown="No Error" w609 {
                  selector: w609 -> [w615 w618]
                  tunnel: [w614 w618] -> w613
                  frame No Error {
                    n223 = call <vilib>:"Error Cluster From Error Code.vi"("error in (no error)"=w615, "error message (\"\")"="SPI port did not reset properly" ("error message (\"\")"), "error code (0)"=-8106) -> ("error out"=w614:errorcluster)  [unwired: 6 in]
                  }
                  frame Error {
                  }
                }
              }
              frame True {
                n224 = call <vilib>:"WPI_SPIRefNum Registry Set.vi"("error in (no error)"=w625, "refnum name"="AutoSPI", "SPIDevRef"=w626) -> ("error out"=w624:errorcluster, "SPIDevRef"=w627:T15)  [unwired: 7 in]
                n225 = call "ADIS16448 Loop Update Status.vi"("ADIS16448 Status"=T16 {"Calibrated?"=FALSE, "IMU Detected?"=TRUE} ("element")) -> ()  [unwired: 10 in, 1 out]
                n226 = Bundle By Name(cluster=w622, "SPIDevRef"=w627, "AutoSPI Active?"=FALSE) -> (w621:T14)
              }
            }
          }
          frame "Start Auto SPI" {
            # "#NOTE Don't do this in register mode."
            n227 = disable-structure shown="Disabled" {
              disable-tunnel: w634 -> [w652 _]
              disable-tunnel: [w643 _] -> w633
              disable-tunnel: w631 -> [w642 _]
              frame Disabled {
                n228 = Unbundle By Name(w642) -> ("SPIDevRef"=w641:T15, "Digital Source"=w640:T8, "ADIS16448DevRef.Hardware Config.Stall Config"=w639:T21, "Data Header"=w638:u8[], "Zero Byte Count"=w637:u8)
                n229 = Unbundle By Name(w641) -> ("SPI Bus"=w653:T6)
                n230 = call <vilib>:"FPGA_SPI_ConfigureAuto.vi"("SPI Auto Zero Byte Count"=w637, "error in"=w652, "SPI Auto TX Byte Array"=w638, "Stall Config"=w639, "SPI Bus"=w653) -> ("error out"=w645:errorcluster)  [unwired: 6 in]
                n231 = call <vilib>:"FPGA_SPI_StartAuto_External.vi"("error in (no error)"=w645, "Falling Edge"=FALSE, "Rising Edge"=TRUE, "Source"=w640) -> ("error out"=w649:errorcluster)  [unwired: 7 in]
                n232 = call <vilib>:"WPI_DigitalOutputRefNum Registry Get.vi"("error in (no error)"=w649, "refnum name"="448 Status LED") -> ("error out"=w648:errorcluster, "DigitalOutputDevRef"=w647:T19)  [unwired: 8 in]
                n233 = call <vilib>:"WPI_DigitalOutputSetValue.vi"("error in (no error)"=w648, "Value"=FALSE, "DigitalOutputDevRef"=w647) -> ("error out"=w643:errorcluster)  [unwired: 7 in, 1 out]
              }
              frame Enabled {
              }
            }
            n234 = RT FIFO Write(0:w635, 1:T18 {"Command"=enum."Recal Complete", "Data"=0} ("element")) -> ()  [unwired: 3 in, 4 out]
            n235 = call <vilib>:"WPI_UtilitiesFRC SendMessageToConsole.vi"("Message"="ADIS16448 Alt start auto SPI requested" ("format string")) -> ()  [unwired: 14 in, 1 out]
          }
          frame "Start Recal" {
            n236 = call "ADIS16448 Loop Update Status.vi"("ADIS16448 Status"=T16 {"Calibrated?"=FALSE, "IMU Detected?"=TRUE} ("element")) -> ()  [unwired: 10 in, 1 out]
            n237 = RT FIFO Write(0:w655, 1:T18 {"Command"=enum."Recalibrate", "Data"=0} ("element")) -> ()  [unwired: 3 in, 4 out]
            n238 = disable-structure shown="Disabled" {
              frame Disabled {
                n239 = call <vilib>:"WPI_UtilitiesFRC SendMessageToConsole.vi"("Message"="ADIS16448 Alt start recal requested" ("format string")) -> ()  [unwired: 14 in, 1 out]
              }
              frame Enabled {
              }
            }
          }
          frame "Configure Cal" {
            n240 = disable-structure shown="Disabled" {
              frame Disabled {
                n241 = call <vilib>:"WPI_UtilitiesFRC SendMessageToConsole.vi"("Message"="ADIS16448 Alt config cal reqeusted" ("format string")) -> ()  [unwired: 14 in, 1 out]
              }
              frame Enabled {
              }
            }
            n242 = Multiply(x=w661, y=u32 100) -> (x*y=w662:u32)
            n243 = Bundle By Name(cluster=w666, "ADIS16448DevRef.Calibration Time"=w661, "CalSamplesAlt"=w662) -> (w665:T14)
          }
        }
      }
      frame "Cal_Init_Alt" {
        n244 = Unbundle By Name(w676) -> ("ADIS16448DevRef.Calibration Time"=w675:u32)
        n245 = Multiply(x=w675, y=u32 100) -> (x*y=w673:u32)
        n246 = Bundle By Name(cluster=w676, "CalSamplesAlt"=w673, "CalCountAlt"=0) -> (w669:T14)
      }
      frame "Cal_Alt" {
        # "read registers one at a time...."
        n247 = Unbundle By Name(w687) -> ("SPIDevRef"=w704:T15, "CalSamplesAlt"=w688:i32, "CalCountAlt"=w699:i32, "Offsets"=w680:dbl[], "Data"=w679:dbl[], "Reset"=w678:bool)
        n248 = for {
          tunnel: w689 -> [w722] mode=indexing
          shift-right: [w715] -> w703
          shift-left: w702 -> [w719]
          shift-right: [w710] -> _
          shift-left: w704 -> [w721]
          shift-right: [w711] -> w693
          shift-left: w695 -> [w718]
          # "hi\nlow"
          n249 = Unbundle(w722) -> ("Reg"=w720:T12, "Data"=w717:u16)
          n250 = call "ADIS16448 Read Register.vi"("error in (no error)"=w719, "ADIS16448 Register"=w720, "SPIDevRef in"=w721) -> ("error out"=w715:errorcluster, "Register Value"=w714:u16, "SPIDevRef out"=w710:T15)  [unwired: 6 in]
          n251 = Increment(x=w717) -> (x+1=w716:u16)
          n252 = Split Number(x=w714) -> (hi(x)=w713:u8, lo(x)=w712:u8)
          n253 = Replace Array Subset(array=w718, new element #1=w713, index #1=w717, new element #2=w712, index #2=w716) -> (w711:u8[])
        }
        n254 = call <vilib>:"Util_GetTime.vi"() -> ("FPGA_Time_Seconds"=w692:dbl)  [unwired: 10 in, 1 out]
        n255 = call "ADIS16448 Scale Data_Alt.vi"("error in (no error)"=w703, "New Data In"=w693) -> ("error out"=w683:errorcluster, "Data Out"=w684:dbl[])  [unwired: 7 in, 1 out]
        n256 = feedback #3(w692) -> (w691:dbl)
        n257 = feedback-in #3(w692) -> ()
        n258 = call "ADIS16448 Loop Manage Cal Buffer.vi"("Sample Count"=w688, "Data In"=w684) -> ()  [unwired: 9 in, 1 out]
        n259 = Subtract(x=w692, y=w691) -> (x-y=w690:dbl)
        n260 = Increment(x=w699) -> (x+1=w700:i32)
        n261 = Greater?(x=w699, y=w688) -> (0:w694:bool)
        n262 = global write "ADIS16448 Globals.vi" "Calibration Count"(w700) -> ()
        n263 = call "ADIS16448 Loop Post Scale.vi"("TimePeriod"=w690, "Reset"=w678, "Data In"=w679, "Offsets"=w680, "Scaled Data In"=w684) -> ("Reset Out"=w681:bool, "Data Out"=w682:dbl[])  [unwired: 5 in]
        n264 = Bundle By Name(cluster=w687, "CalCountAlt"=w700, "Data"=w682, "Reset"=w681) -> (w685:T14)
        n265 = Wait (ms)(milliseconds to wait=u32 10) -> ()  [unwired: 1 out]
        n266 = case shown="True" w694 {
          tunnel: w685 -> [w705 w706]
          tunnel: [w705 w707] -> w686
          frame False {
          }
          frame True {
            n267 = call "ADIS16448 Loop Manage Cal Buffer.vi"("Cmd"=ADIS16448_Call_Buffer_Cmd."Calculate") -> ("Cal Offset Out"=w708:dbl[])  [unwired: 10 in]
            n268 = Bundle By Name(cluster=w706, "Offsets"=w708) -> (w707:T14)
            n269 = global write "ADIS16448 Globals.vi" "CallOffsets"(w708) -> ()
          }
        }
        n270 = Select(t=ADIS16448_Loop_State."Finish Cal", s=w694, f=ADIS16448_Loop_State."Cal_Alt") -> (s? t:f=w698:T13)
      }
    }
  }
  n271 = Open VI Reference(vi path="Main Name") -> (vi reference=w22:refnum<vi>)  [unwired: 3 in, 3 out]
  n272 = while {
    tunnel: w22 -> [w724]
    tunnel: [w723] -> w15
    stop <- w723 stop-if-true
    # "stop this VI when the VI calling StartComm goes idle"
    n273 = property class="VI"(reference=w724) -> ("Exec.State"=w726:T23)  [unwired: 1 in, 2 out]
    n274 = Wait (ms)(milliseconds to wait=u32 250) -> ()  [unwired: 1 out]
    n275 = Equal?(x=w726, y=T23."Idle" ("Execution:State")) -> (x = y?=w723:bool)
  }
  n276 = flat-sequence {
    tunnel: w15 -> [_]
    frame #0 {
      n277 = call <vilib>:"WPI_DigitalOutputRefNum Registry Get.vi"("refnum name"="448 Status LED") -> ("error out"=w733:errorcluster, "DigitalOutputDevRef"=w732:T19)  [unwired: 9 in]
      n278 = call <vilib>:"WPI_DigitalOutputClose.vi"("error in (no error)"=w733, "DigitalOutputDevRef"=w732) -> ("error out"=w728:errorcluster)  [unwired: 9 in]
      n279 = call <vilib>:"WPI_SPIRefNum Registry Get.vi"("error in (no error)"=w728, "refnum name"="AutoSPI") -> ("error out"=w730:errorcluster, "SPIDevRef"=w729:T15)  [unwired: 8 in]
      n280 = call <vilib>:"WPI_SPIClose.vi"("error in (no error)"=w730, "SPIDevRef"=w729) -> ()  [unwired: 9 in, 1 out]
    }
    frame #1 {
      n281 = Stop() -> ()  [unwired: 1 in]
    }
  }
  n282 = flat-sequence {
    tunnel: w15 -> [_]
    frame #0 {
      # "#NOTE JAS Added .... never called.."
      n283 = call <vilib>:"WPI_UtilitiesFRC SendMessageToConsole.vi"("Message"="ADIS16448 Processing loop terminating." ("format string")) -> ()  [unwired: 14 in, 1 out]
    }
  }
